vi "contrl.vi"() -> ()   [LabVIEW 2015]
uses:
  Ctrls/Main vari.ctl
  Mode/config/CHS.ctl
  Mode/config/singlechtype.ctl
  Ctrls/command.ctl
  TCPIP/TCPIP_enum.ctl
  TCPIP/TCPIPconfig.ctl
panel:
  out "P34 2":dbl
  in  "command":T1=22 items=["NO_Action", "start", "pause", "resum", "stop", "config", "System_constant", "7", "DAQ_init", "DAQ_config", "DAQ_start", "DAQ_read", "DAQ_stop", "DAQ_contrl", "14", "15", "16", "17", "18", "19", "Zsf_open", "Zsf_close", "Wkf_control", "Pump_switch", "dcf_switch", "JRQ_switch"]
  out "error out":errorcluster
  out "LED":bool[](array[boolean])
  in  "Tab Control":enum32{"核心舱", "实验舱", "温度曲线", "压力曲线", "内回路"}(tab)
  out "temp1 2":dbl(slide) caption="液温2" scale=0.0..100.0 scale format="%#_6f"
  out "temp2 2":dbl(slide) caption="液温1" scale=0.0..100.0 scale format="%.1f"
  out "PT22":dbl format="%#.1f"
  out "PT23":dbl
  out "转速":dbl format="%#.1f"
  out "流量计 2":dbl(knob) scale=0.0..1800.0 scale format="%#_6f"
  out "P34":dbl
  out "T4":dbl format="%#.1f"
  out "温控阀a":dbl(knob) scale=-10.0..60.0 scale format="%#.2f"
  out "zsf12":bool
  out "zsf11":bool
  out "zsf10":bool
  out "zsf9":bool
  out "zsf8":bool
  out "zsf7":bool
  out "zsf6":bool
  out "zsf5":bool
  out "zsf4":bool
  out "zsf3":bool
  out "zsf2":bool
  out "zsf1":bool
  in  "temctr_run 2":bool
  in  "temctr_value 2":dbl caption="设置"
  in  "temctr_type 2":enum16{"开度", "控温"}(ring)
  out "unit":string
  in  "temctr_run":bool
  in  "temctr_type":enum16{"开度", "控温"}(ring)
  in  "WP":bool
  in  "ZP":bool
  in  "rlmn 4":bool caption="加热模拟"
  in  "rlmn 3":bool caption="加热模拟"
  in  "rlmn 5":bool caption="加热模拟"
  out "PT21":dbl format="%#.1f"
  out "T2":dbl format="%#.1g"
  out "T22":dbl format="%#.1f"
  out "T1":dbl format="%#.1f"
  out "PT2":dbl format="%#.1f"
  out "T3":dbl format="%#.1f"
  out "T4":dbl format="%#.1f"
  out "PT3":dbl format="%#.1f"
  out "PT1":dbl format="%#.1f"
  out "P19":dbl format="%#.1f"
  out "P18":dbl format="%#.1f"
  out "P17":dbl format="%#.1g"
  out "P16":dbl format="%#.1f"
  out "P15":dbl format="%#.1f"
  out "P14":dbl format="%#.1f"
  out "P13":dbl format="%#.1f"
  out "P12":dbl format="%#.1f"
  out "DP2":dbl format="%#.2f"
  out "P11":dbl
  out "P10":dbl
  out "PT15":dbl
  out "PT16":dbl
  out "PT13":dbl
  out "PT14":dbl
  out "DP1":dbl format="%#.2g"
  out "P9":dbl format="%#.1f"
  out "P35":dbl format="%#.1f"
  out "P10":dbl format="%#.1f"
  out "P16":dbl format="%#.1f"
  out "P15":dbl format="%#.1f"
  out "P14":dbl format="%#.1f"
  out "P13":dbl format="%#.1f"
  out "P12":dbl format="%#.1f"
  out "P11":dbl format="%#.1f"
  out "T1":dbl format="%#.1f"
  out "PT8":dbl format="%#.1f"
  out "T2":dbl format="%#.1f"
  out "PT2":dbl format="%#.1f"
  out "PT1":dbl format="%#.2g"
  out "PT3":dbl format="%#.1f"
  out "T3":dbl format="%#.1f"
  out "PT4":dbl format="%#.1f"
  out "PT7":dbl format="%#.1f"
  out "PT9":dbl format="%#.1f"
  out "PT5":dbl format="%#.1f"
  out "ZF16":bool
  out "ZF17":bool
  in  "DCF19":bool
  in  "DCF18":bool
  in  "DCF17":bool
  in  "DCF16":bool
  in  "DCF15":bool
  in  "DCF14":bool
  in  "DCF13":bool
  in  "DCF12":bool
  in  "DCF11":bool
  in  "DCF10":bool
  in  "DCF9":bool
  in  "DCF8":bool
  out "DG8":bool
  out "DG7":bool
  out "DG6":bool
  out "DG5":bool
  out "G321":bool
  out "DG166":bool
  in  "qyflq 3":bool caption="气液分离器 3"
  out "ZF14":bool
  out "补偿器":dbl(slide) scale=0.0..200.0
  out "ZF13":bool
  out "G1114":bool
  out "G115":bool
  out "G131":bool
  out "G142":bool
  out "G112":bool
  out "G132":bool
  out "G133":bool
  out "G133":bool(c317)
  in  "DCF6":bool
  in  "DCF7":bool
  out "G113":bool
  in  "DCF5":bool
  out "G135":bool
  out "G134":bool
  out "G111":bool
  in  "DCF4":bool
  out "G141":bool
  out "流量计":dbl(knob) scale=0.0..1800.0 scale format="%#_6f"
  out "G181":bool
  out "G191":bool
  out "G201":bool
  out "补偿器":dbl(slide) scale=0.0..150.0 scale format="%#.1f"
  in  "DCF3":bool
  in  "DCF2":bool
  in  "DCF1":bool
  out "G999":bool
  out "G998":bool
  out "G401":bool
  out "G60":bool
  out "G58":bool
  out "G56":bool
  out "G53":bool
  out "G51":bool
  out "G49":bool
  out "G47":bool
  out "G45":bool
  out "G42":bool
  out "G61":bool
  out "G52":bool
  out "G54":bool
  out "G1313":bool
  out "G1312":bool
  out "G1311":bool
  out "G1310":bool
  out "G139":bool
  out "G138":bool
  out "G137":bool
  out "G136":bool
  in  "fsq6":bool caption="辐射器"
  in  "fsq5":bool caption="辐射器"
  in  "fsq4":bool caption="辐射器"
  in  "fsq3":bool caption="辐射器"
  in  "fsq2":bool caption="辐射器"
  out "G135":bool
  out "G134":bool
  out "G133":bool
  out "G132":bool
  out "G59":bool
  out "G57":bool
  out "G55":bool
  out "G43":bool
  out "G50":bool
  out "G48":bool
  out "G46":bool
  out "G44":bool
  out "G41":bool
  in  "ZSF12":bool
  in  "ZSF11":bool
  in  "ZSF10":bool
  in  "ZSF09":bool
  in  "ZSF08":bool
  in  "ZSF07":bool
  in  "ZSF06":bool
  in  "ZSF05":bool
  in  "ZSF04":bool
  in  "ZSF03":bool
  in  "ZSF02":bool
  out "G40":bool
  in  "ZSF01":bool
  in  "辐射器":bool
  out "电压":dbl
  out "电流":dbl
  out "转速":dbl
  out "DG11":bool
  out "ZF12":bool
  out "DG9":bool
  in  "DG4":bool
  in  "rlmn2":bool caption="加热模拟"
  out "DG3":bool
  in  "qyflq2":bool caption="气液分离器 2"
  out "ZF11":bool
  out "DG2":bool
  out "pumpD":bool
  out "ZG31":bool
  out "ZG14":bool
  out "ZF10":bool
  out "ZF9":bool
  out "ZF8":bool
  out "ZF7":bool
  out "ZF6":bool
  out "ZG8 2":bool
  out "ZF5":bool
  out "ZF4":bool
  out "ZF3":bool
  in  "qyflq":bool
  out "ZG8":bool
  out "ZF2":bool
  out "ZF1":bool
  out "ZG6":bool
  out "ZG30":bool
  out "ZG27":bool
  out "ZG24":bool
  out "ZG25":bool
  out "ZG26":bool
  out "ZG23":bool
  out "ZG22":bool
  out "ZG21":bool
  out "ZG20":bool
  out "ZG19":bool
  out "ZG18":bool
  out "ZG16":bool
  out "ZG15":bool
  out "ZG17":bool
  out "ZG13":bool
  in  "Zyshj":bool caption="视液镜"
  in  "ysj":bool caption="视液镜"
  out "ZG12":bool
  out "ZG11":bool
  out "ZG10":bool
  out "ZG9":bool
  out "ZG7":bool
  out "ZG5":bool
  out "ZG4":bool
  out "ZG3":bool
  out "ZG2":bool
  out "G38":bool
  out "ZG1":bool(c317)
  out "DG1":bool(c317)
  in  "rlmn１":bool caption="热量模拟"
  in  "yzmn":bool caption="液阻模拟"
  out "G37":bool
  out "G36":bool
  out "G34":bool
  out "G35":bool
  out "G30":bool(c317)
  out "温控阀ｂ":dbl(knob) scale=-10.0..60.0 scale format="%#.2g"
  out "G32":bool
  out "G31":bool
  out "SF2 2":bool
  out "G33":bool
  out "G29":bool
  out "G28":bool
  out "G27":bool
  out "temp1":dbl(slide) caption="液温2" scale=0.0..100.0 scale format="%#_6f"
  out "temp2":dbl(slide) caption="液温1" scale=0.0..100.0 scale format="%.1f"
  out "G25":bool
  out "G24":bool
  out "G23":bool
  out "G22":bool
  out "G21":bool
  out "G20":bool
  out "G19":bool
  out "G18":bool
  out "G17":bool
  out "G16":bool
  out "G15":bool
  out "G14":bool
  out "SF2":bool
  out "G13":bool
  out "pump":bool caption="外回路泵"
  out "G12":bool
  out "G11":bool
  out "G10":bool
  out "G9":bool
  out "G8":bool
  out "G7":bool
  out "G6":bool
  out "G4":bool
  out "G5":bool
  out "G3":bool
  out "pumpZ":bool caption="中温内回路泵"
  out "DG10":bool
  out "G2":bool
  out "SF1":bool
  out "wkf1":dbl caption="值" format="%#.1f"
  in  "temctr_value":dbl caption="设置"
  out "wkf2":dbl caption="值" format="%#.2g"
  out "temp1 4":dbl(slide) caption="液温2" scale=0.0..100.0 scale format="%#_6f"
  out "temp2 4":dbl(slide) caption="液温1" scale=0.0..100.0 scale format="%.1f"
  out "PT22 2":dbl format="%#.1f"
  out "PT23 2":dbl
  out "转速  3":dbl format="%#.1f"
  out "T4 3":dbl caption="T4" format="%#.1f"
  out "实验舱温控阀a":dbl(knob) caption="温控阀a" scale=-10.0..60.0 scale format="%#.2f"
  in  "temctr_run 4":bool
  in  "temctr_value 4":dbl caption="设置"
  in  "temctr_type 4":enum16{"开度", "控温"}(ring)
  out "unit 2":string
  in  "temctr_run 3":bool
  in  "temctr_type 3":enum16{"开度", "控温"}(ring)
  in  "WP 2":bool
  in  "ZP 2":bool
  in  "rlmn 8":bool caption="加热模拟"
  in  "rlmn 7":bool caption="加热模拟"
  in  "rlmn 6":bool caption="加热模拟"
  out "PT21 2":dbl format="%#.1f"
  out "T2 3":dbl format="%#.1g"
  out "T22 2":dbl format="%#.1f"
  out "T1 3":dbl format="%#.1f"
  out "PT2 3":dbl format="%#.1f"
  out "T3 3":dbl format="%#.1f"
  out "T4 2":dbl format="%#.1f"
  out "PT3 3":dbl format="%#.1f"
  out "PT1 3":dbl format="%#.1f"
  out "P19syc":dbl caption="内压传感器" format="%#.1f"
  out "P18 2":dbl format="%#.1f"
  out "P17 2":dbl format="%#.1g"
  out "P16 3":dbl format="%#.1f"
  out "P15 3":dbl format="%#.1f"
  out "P14 3":dbl format="%#.1f"
  out "P13 3":dbl format="%#.1f"
  out "P12 3":dbl format="%#.1f"
  out "DP2 2":dbl format="%#.2f"
  out "P11 3":dbl
  out "P10 3":dbl
  out "PT15 2":dbl
  out "PT16 2":dbl
  out "PT13 2":dbl
  out "PT14 2":dbl
  out "DP_syc":dbl caption="DP" format="%#.2g"
  out "syP9":dbl caption="外压2" format="%#.1f"
  out "syP35":dbl caption="外压3" format="%#.1f"
  out "P10_syc":dbl format="%#.1f"
  out "T1_syc":dbl caption="T1" format="%#.1f"
  out "PT8 2":dbl format="%#.1f"
  out "T2 2":dbl format="%#.1f"
  out "PT2 2":dbl format="%#.1f"
  out "PT1 2":dbl format="%#.2g"
  out "PT3 2":dbl format="%#.1f"
  out "T3 2":dbl format="%#.1f"
  out "PT4 2":dbl format="%#.1f"
  out "PT7 2":dbl format="%#.1f"
  out "PT9 2":dbl format="%#.1f"
  out "PT5 2":dbl format="%#.1f"
  out "ZF16 2":bool
  out "ZF17 2":bool
  out "DG8 2":bool
  out "DG7 2":bool
  out "DG6 2":bool
  out "DG5 2":bool
  out "G321 2":bool
  out "DG166 2":bool
  in  "qyflq 4":bool caption="气液分离器 3"
  out "ZF14 2":bool
  out "补偿器_sycw":dbl(slide) scale=0.0..200.0
  out "ZF13 2":bool
  out "G112 2":bool
  out "G132 3":bool
  out "G133 4":bool
  out "G133 3":bool(c317)
  out "G113 2":bool
  out "G135 3":bool
  out "G134 3":bool
  out "G111 2":bool
  out "G141 2":bool
  out "补偿器 2":dbl(slide) scale=0.0..150.0 scale format="%#.1f"
  out "G999 2":bool
  out "G998 2":bool
  out "G401 2":bool
  out "G60 2":bool
  out "G58 2":bool
  out "G56 2":bool
  out "G53 2":bool
  out "G51 2":bool
  out "G49 2":bool
  out "G47 2":bool
  out "G45 2":bool
  out "G42 2":bool
  out "G61 2":bool
  out "G52 2":bool
  out "G54 2":bool
  out "G1313 2":bool
  out "G1312 2":bool
  out "G1311 2":bool
  out "G1310 2":bool
  out "G139 2":bool
  out "G138 2":bool
  out "G137 2":bool
  out "G136 2":bool
  in  "fsq6 2":bool caption="辐射器"
  in  "fsq5 2":bool caption="辐射器"
  in  "fsq4 2":bool caption="辐射器"
  in  "fsq3 2":bool caption="辐射器"
  in  "fsq2 2":bool caption="辐射器"
  out "G135 2":bool
  out "G134 2":bool
  out "G133 2":bool
  out "G132 2":bool
  out "G59 2":bool
  out "G57 2":bool
  out "G55 2":bool
  out "G43 2":bool
  out "G50 2":bool
  out "G48 2":bool
  out "G46 2":bool
  out "G44 2":bool
  out "G41 2":bool
  out "G40 2":bool
  in  "辐射器 2":bool
  out "电压 2":dbl
  out "电流 2":dbl
  out "转速 2":dbl
  out "DG11 2":bool
  out "ZF12 2":bool
  out "DG9 2":bool
  in  "DG4 2":bool
  in  "rlmn2 2":bool caption="加热模拟"
  out "DG3 2":bool
  in  "qyflq2 2":bool caption="气液分离器 2"
  out "ZF11 2":bool
  out "DG2 2":bool
  out "pumpD 2":bool
  out "ZG31 2":bool
  out "ZG14 2":bool
  out "ZF10 2":bool
  out "ZF9 2":bool
  out "ZF8 2":bool
  out "ZF7 2":bool
  out "ZF6 2":bool
  out "ZG8 4":bool
  out "ZF5 2":bool
  out "ZF4 2":bool
  out "ZF3 2":bool
  in  "qyflq 2":bool
  out "ZG8 3":bool
  out "ZF2 2":bool
  out "ZF1 2":bool
  out "ZG6 2":bool
  out "ZG30 2":bool
  out "ZG27 2":bool
  out "ZG24 2":bool
  out "ZG25 2":bool
  out "ZG26 2":bool
  out "ZG23 2":bool
  out "ZG22 2":bool
  out "ZG21 2":bool
  out "ZG20 2":bool
  out "ZG19 2":bool
  out "ZG18 2":bool
  out "ZG16 2":bool
  out "ZG15 2":bool
  out "ZG17 2":bool
  out "ZG13 2":bool
  in  "Zyshj 2":bool caption="视液镜"
  in  "ysj 2":bool caption="视液镜"
  out "ZG12 2":bool
  out "ZG11 2":bool
  out "ZG10 2":bool
  out "ZG9 2":bool
  out "ZG7 2":bool
  out "ZG5 2":bool
  out "ZG4 2":bool
  out "ZG3 2":bool
  out "ZG2 2":bool
  out "G38 2":bool
  out "ZG1 2":bool(c317)
  out "DG1 2":bool(c317)
  in  "rlmn１ 2":bool caption="热量模拟"
  in  "yzmn 2":bool caption="液阻模拟"
  out "G37 2":bool
  out "G36 2":bool
  out "G34 2":bool
  out "G35 2":bool
  out "G30 2":bool(c317)
  out "温控阀ｂ 2":dbl(knob) scale=-10.0..60.0 scale format="%#.2g"
  out "G32 2":bool
  out "G31 2":bool
  out "SF2 4":bool
  out "G33 2":bool
  out "G29 2":bool
  out "G28 2":bool
  out "G27 2":bool
  out "temp1 3":dbl(slide) caption="液温2" scale=0.0..100.0 scale format="%#_6f"
  out "temp2 3":dbl(slide) caption="液温1" scale=0.0..100.0 scale format="%.1f"
  out "G25 2":bool
  out "G24 2":bool
  out "G23 2":bool
  out "G22 2":bool
  out "G21 2":bool
  out "G20 2":bool
  out "G19 2":bool
  out "G18 2":bool
  out "G17 2":bool
  out "G16 2":bool
  out "G15 2":bool
  out "G14 2":bool
  out "SF2 3":bool
  out "G13 2":bool
  out "pump 2":bool caption="外回路泵"
  out "G12 2":bool
  out "G11 2":bool
  out "G10 2":bool
  out "G9 2":bool
  out "G8 2":bool
  out "G7 2":bool
  out "G6 2":bool
  out "G4 2":bool
  out "G5 2":bool
  out "G3 2":bool
  out "pumpZ 2":bool caption="中温内回路泵"
  out "DG10 2":bool
  out "G2 2":bool
  out "SF1 2":bool
  out "wkf1 2":dbl caption="值" format="%#.1f"
  in  "temctr_value 3":dbl caption="设置"
  out "wkf2 2":dbl caption="值" format="%#.2g"
  out "测试数据":string[][](table)
  out "T Wave":dbl[](graph) caption="Vibr Wave"
  out "XY Graph":cluster{cluster{"time":dbl, "Y":dbl}[]}[](graph)
  out "Vibr Wave 3":dbl[](graph) caption="Vibr Wave"
  out "triger?":bool caption="采集\n触发"
  out "save":bool caption="数据\n存储"
  in  "Query":bool
  in  "Exit":bool
  in  "Acquire":bool
  in  "Config":bool
  in  "Vibr Waveform 2":waveform(dbl)[](array[waveform])
  out "throber 2":bool
  in  "Main Vari":T2={"Error"={"status"=FALSE, "code"=0, "source"=""}, "Test Info"={"Test Name"="", "Tester"=""}, "StateName"="", "Display Info"=[{"Frequency"=0.0, "RMS"=0.0}, {"Frequency"=0.0, "RMS"=0.0}, {"Frequency"=0.0, "RMS"=0.0}, {"Frequency"=0.0, "RMS"=0.0}, {"Frequency"=0.0, "RMS"=0.0}], "粉尘特性"={"名称"="", "粒径"="", "含水量"=""}, "测试条件"={"初始含氧量"="", "初始压力"="", "测试浓度"="", "点火能量"="", "初始温度"="", "反应器体积[L]"=0.0}, "ch size"=0, "data out"=[], "CHS"=[], "CalData"=[]} {"CHS"."display" format="%b"}
  # "流体回路多回路试验平台测试系统"
  # "Measurement System Ver 1.0  Copyright  by M_tech design studio"
  # "温控阀控制"
  # "液视镜"
  # "温控阀控制"
  # "液视镜"
  # "通道名称"
  # "颜色"
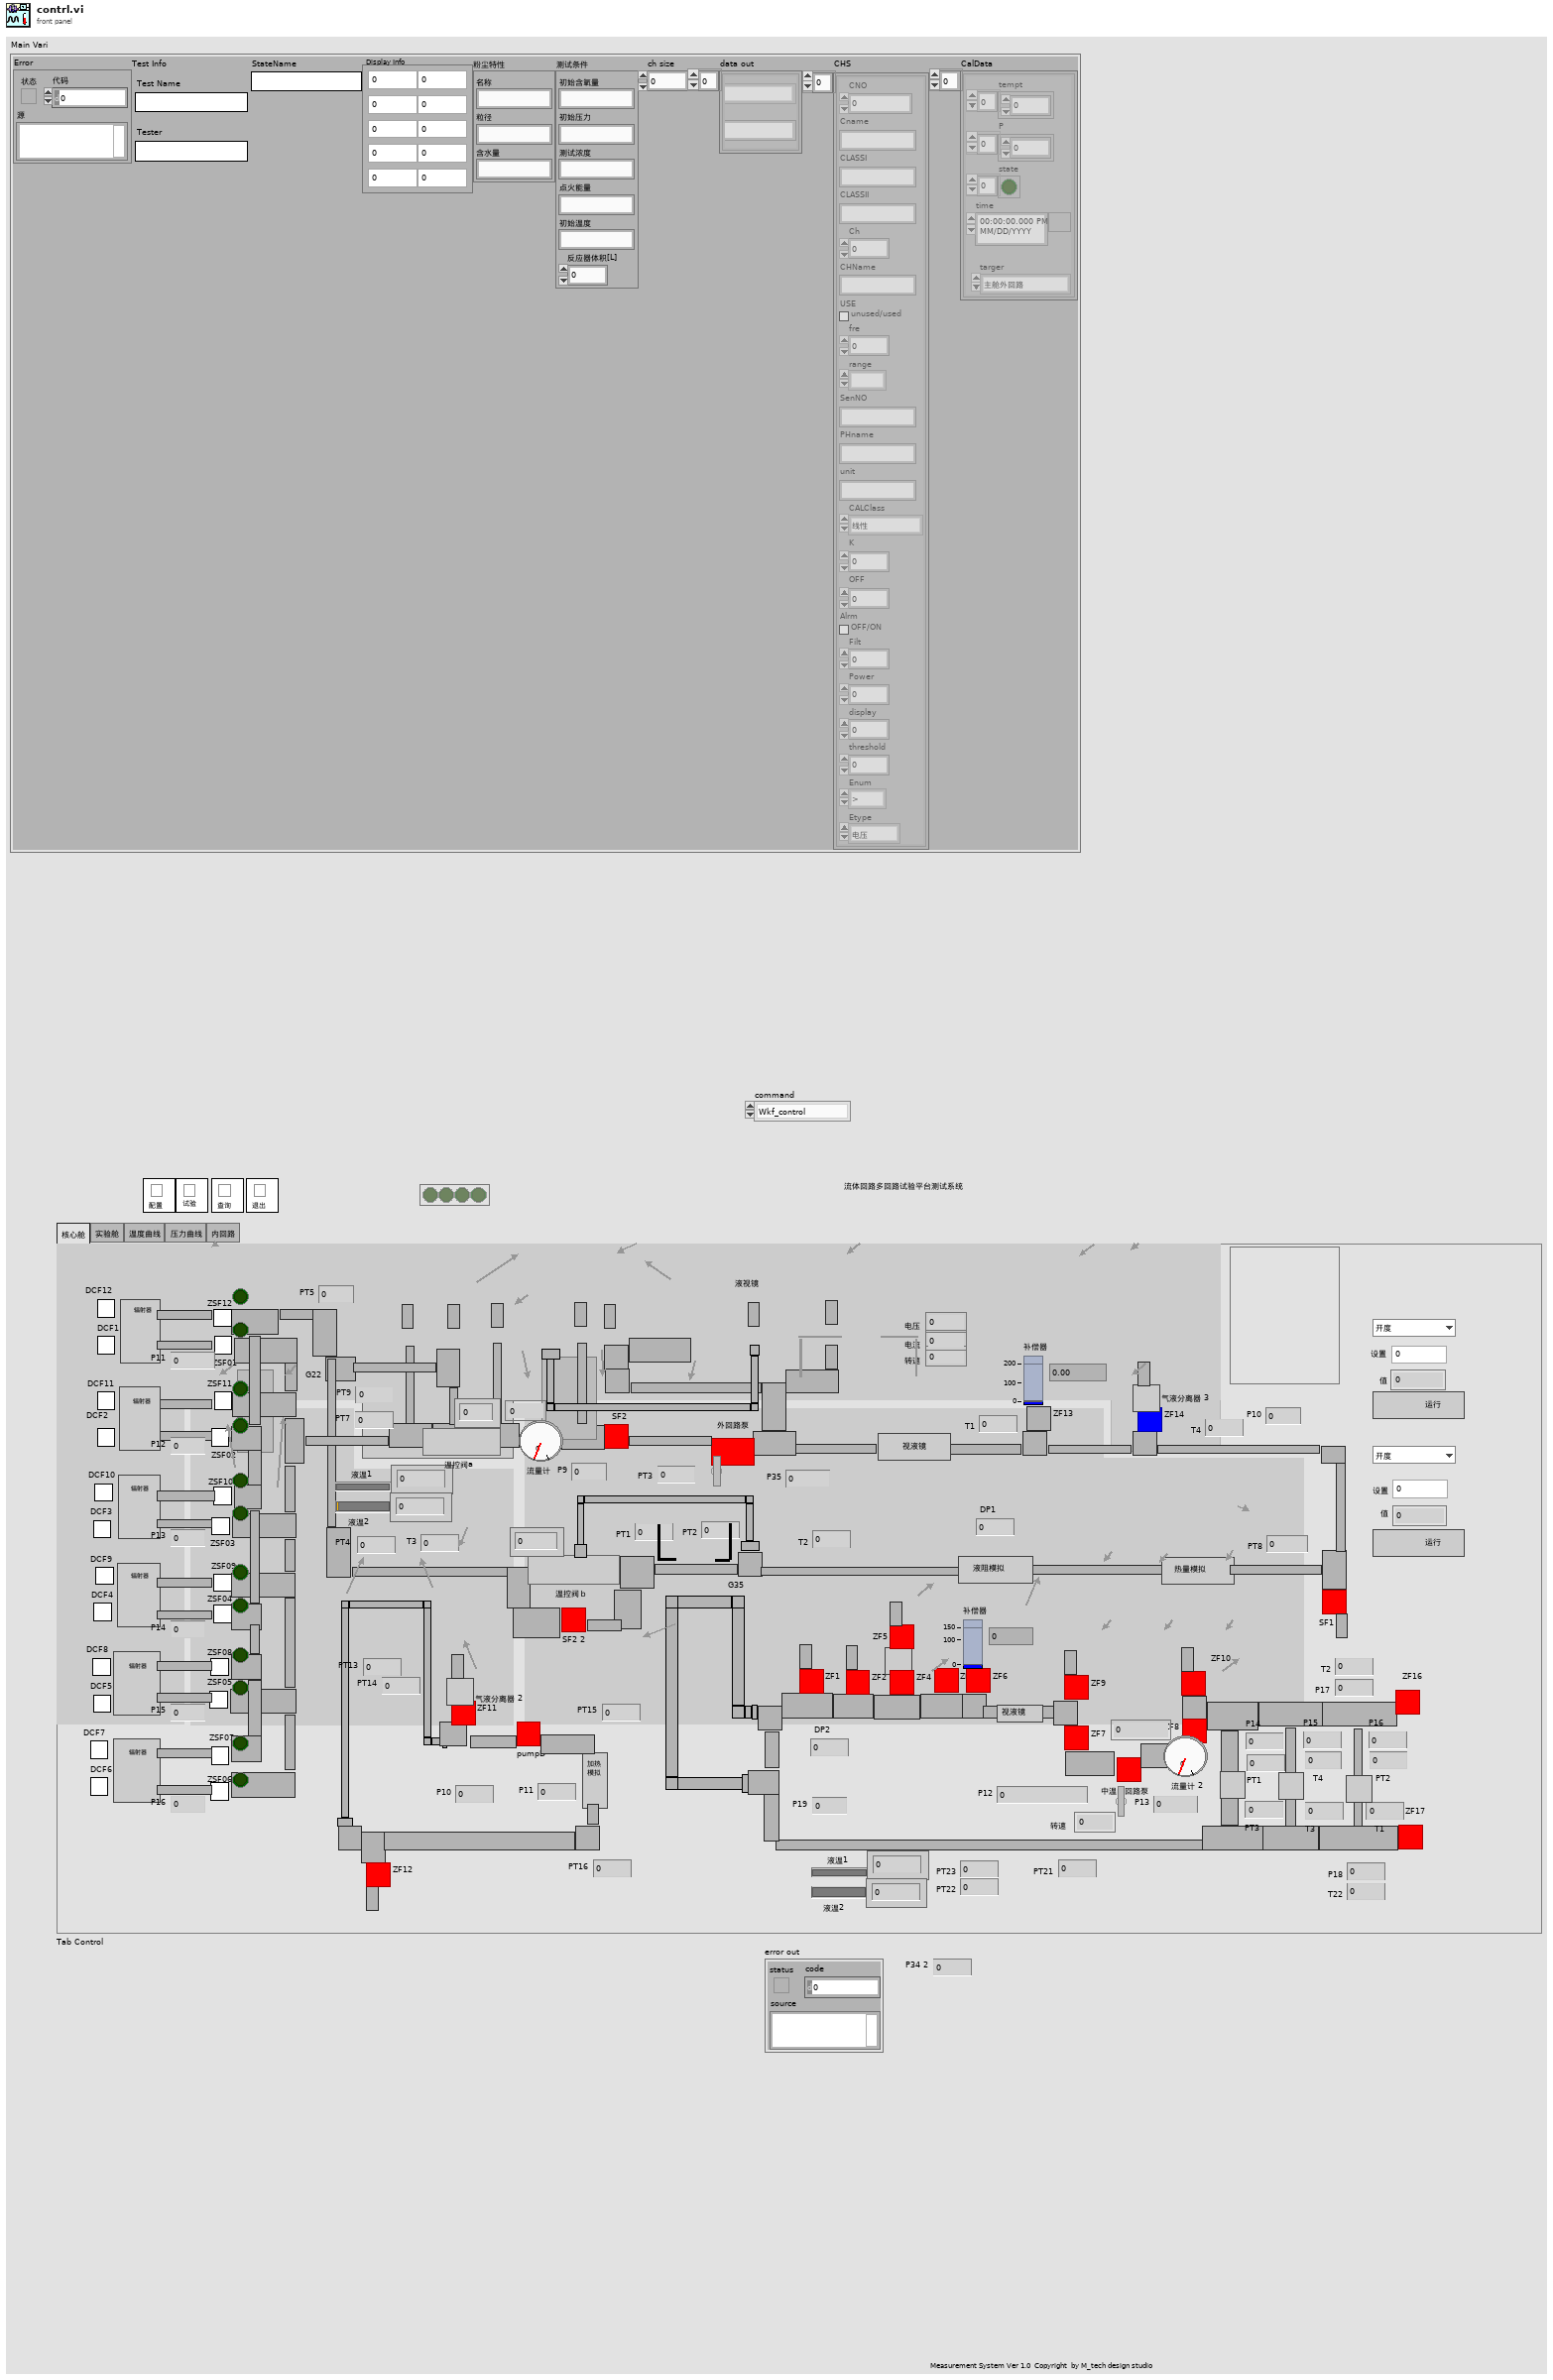
[diagram p1: front panel]
types:
  T1 = typedef "command.ctl" = u16
  T2 = typedef "Main vari.ctl" = cluster{"Error":errorcluster, "Test Info":cluster{"Test Name":string, "Tester":string}, "StateName":string, "Display Info":T3, "粉尘特性":T4, "测试条件":T5, "ch size":u8, "data out":cluster{"targer":enum16{"主舱外回路", "主舱内回路", "实验舱外回路", "实验舱内回路"}, "data":string}[], "CHS":T6, "CalData":cluster{"tempt":dbl[], "P":dbl[], "state":bool[], "time":timestamp, "targer":enum16{"主舱外回路", "主舱内回路", "实验舱外回路", "实验舱内回路"}}[]}
  T3 = typedef "Display Information_Ctrls-某型振动实验台测试系统.ctl" = cluster{"Frequency":dbl, "RMS":dbl}[]
  T4 = typedef "粉尘特性.ctl" = cluster{"名称":string, "粒径":string, "含水量":string}
  T5 = typedef "测试条件.ctl" = cluster{"初始含氧量":string, "初始压力":string, "测试浓度":string, "点火能量":string, "初始温度":string, "反应器体积[L]":dbl}
  T6 = typedef "CHS.ctl" = T7[]
  T7 = typedef "singlechtype.ctl" = cluster{"CNO":u8, "Cname":string, "CLASSI":string, "CLASSII":string, "Ch":u8, "CHName":string, "USE":bool, "fre":dbl, "range":enum16{""}, "SenNO":string, "PHname":string, "unit":string, "CALClass":enum8{"线性", "查表", "公式"}, "K":dbl, "OFF":dbl, "Alrm":bool, "Filt":dbl, "Power":u8, "display":u8, "threshold ":dbl, "Enum":enum16{">", ">=", "<", "<=", "<>(在范围内）", "><（在范围外）"}, "Etype":enum16{"电压", "电流", "电阻", "热电偶K", "热电偶T"}}
  T8 = typedef "Enum queue_Ctrls-某型振动实验台测试系统.ctl" = enum16{"Noop", "Send Pro1", "Send data", "Get Pro1", "Get data", "Flush Pro1", "Flush data", "Destroy Pro1", "Destroy data"}
  T9 = typedef "TCPIPconfig.ctl" = cluster{"add":string, "port":u32, "timeout":u16, "connection ID":refnum<k5>, "targer":enum16{"主舱外回路", "主舱内回路", "实验舱外回路", "实验舱内回路"}}[]
  T10 = cluster{"targer":enum16{"主舱外回路", "主舱内回路", "实验舱外回路", "实验舱内回路"}, "data":string}[]
  T11 = cluster{"targer":enum16{"主舱外回路", "主舱内回路", "实验舱外回路", "实验舱内回路"}, "data":string}
  T12 = typedef "TCPIP_enum.ctl" = enum16{"init", "connect", "command", "write", "read", "close", "null"}
  T13 = cluster{"T":cluster{"TSlop":dbl[], "T0":dbl[]}, "P":cluster{"P0":dbl[], "Pslop":dbl[]}}[]
  T14 = cluster{"T":cluster{"index":dbl, "name":string, "unit":string, "代号":string}[], "P":cluster{"index":dbl, "name":string, "unit":string, "代号":string}[], "state":cluster{"index":dbl, "name":string, "unit":string, "代号":string}[], "time":timestamp, "targer":enum16{"主舱外回路", "主舱内回路", "实验舱外回路", "实验舱内回路"}}[]
  T15 = enum16{"init", "trig", "save", "stop", "Default"}
  T16 = typedef "Enum File IO - FGV(V)_Ctrls-某型振动实验台测试系统.ctl" = enum16{"New", "Open", "Write Info", "Write Data", "Read Info", "Read Chan Names", "Read Data", "Close", "None"}
  T17 = cluster{"tempt":dbl[], "P":dbl[], "state":bool[], "time":timestamp, "targer":enum16{"主舱外回路", "主舱内回路", "实验舱外回路", "实验舱内回路"}}[]
  T18 = cluster{"tempt":dbl[], "P":dbl[], "state":bool[], "time":timestamp, "targer":enum16{"主舱外回路", "主舱内回路", "实验舱外回路", "实验舱内回路"}}
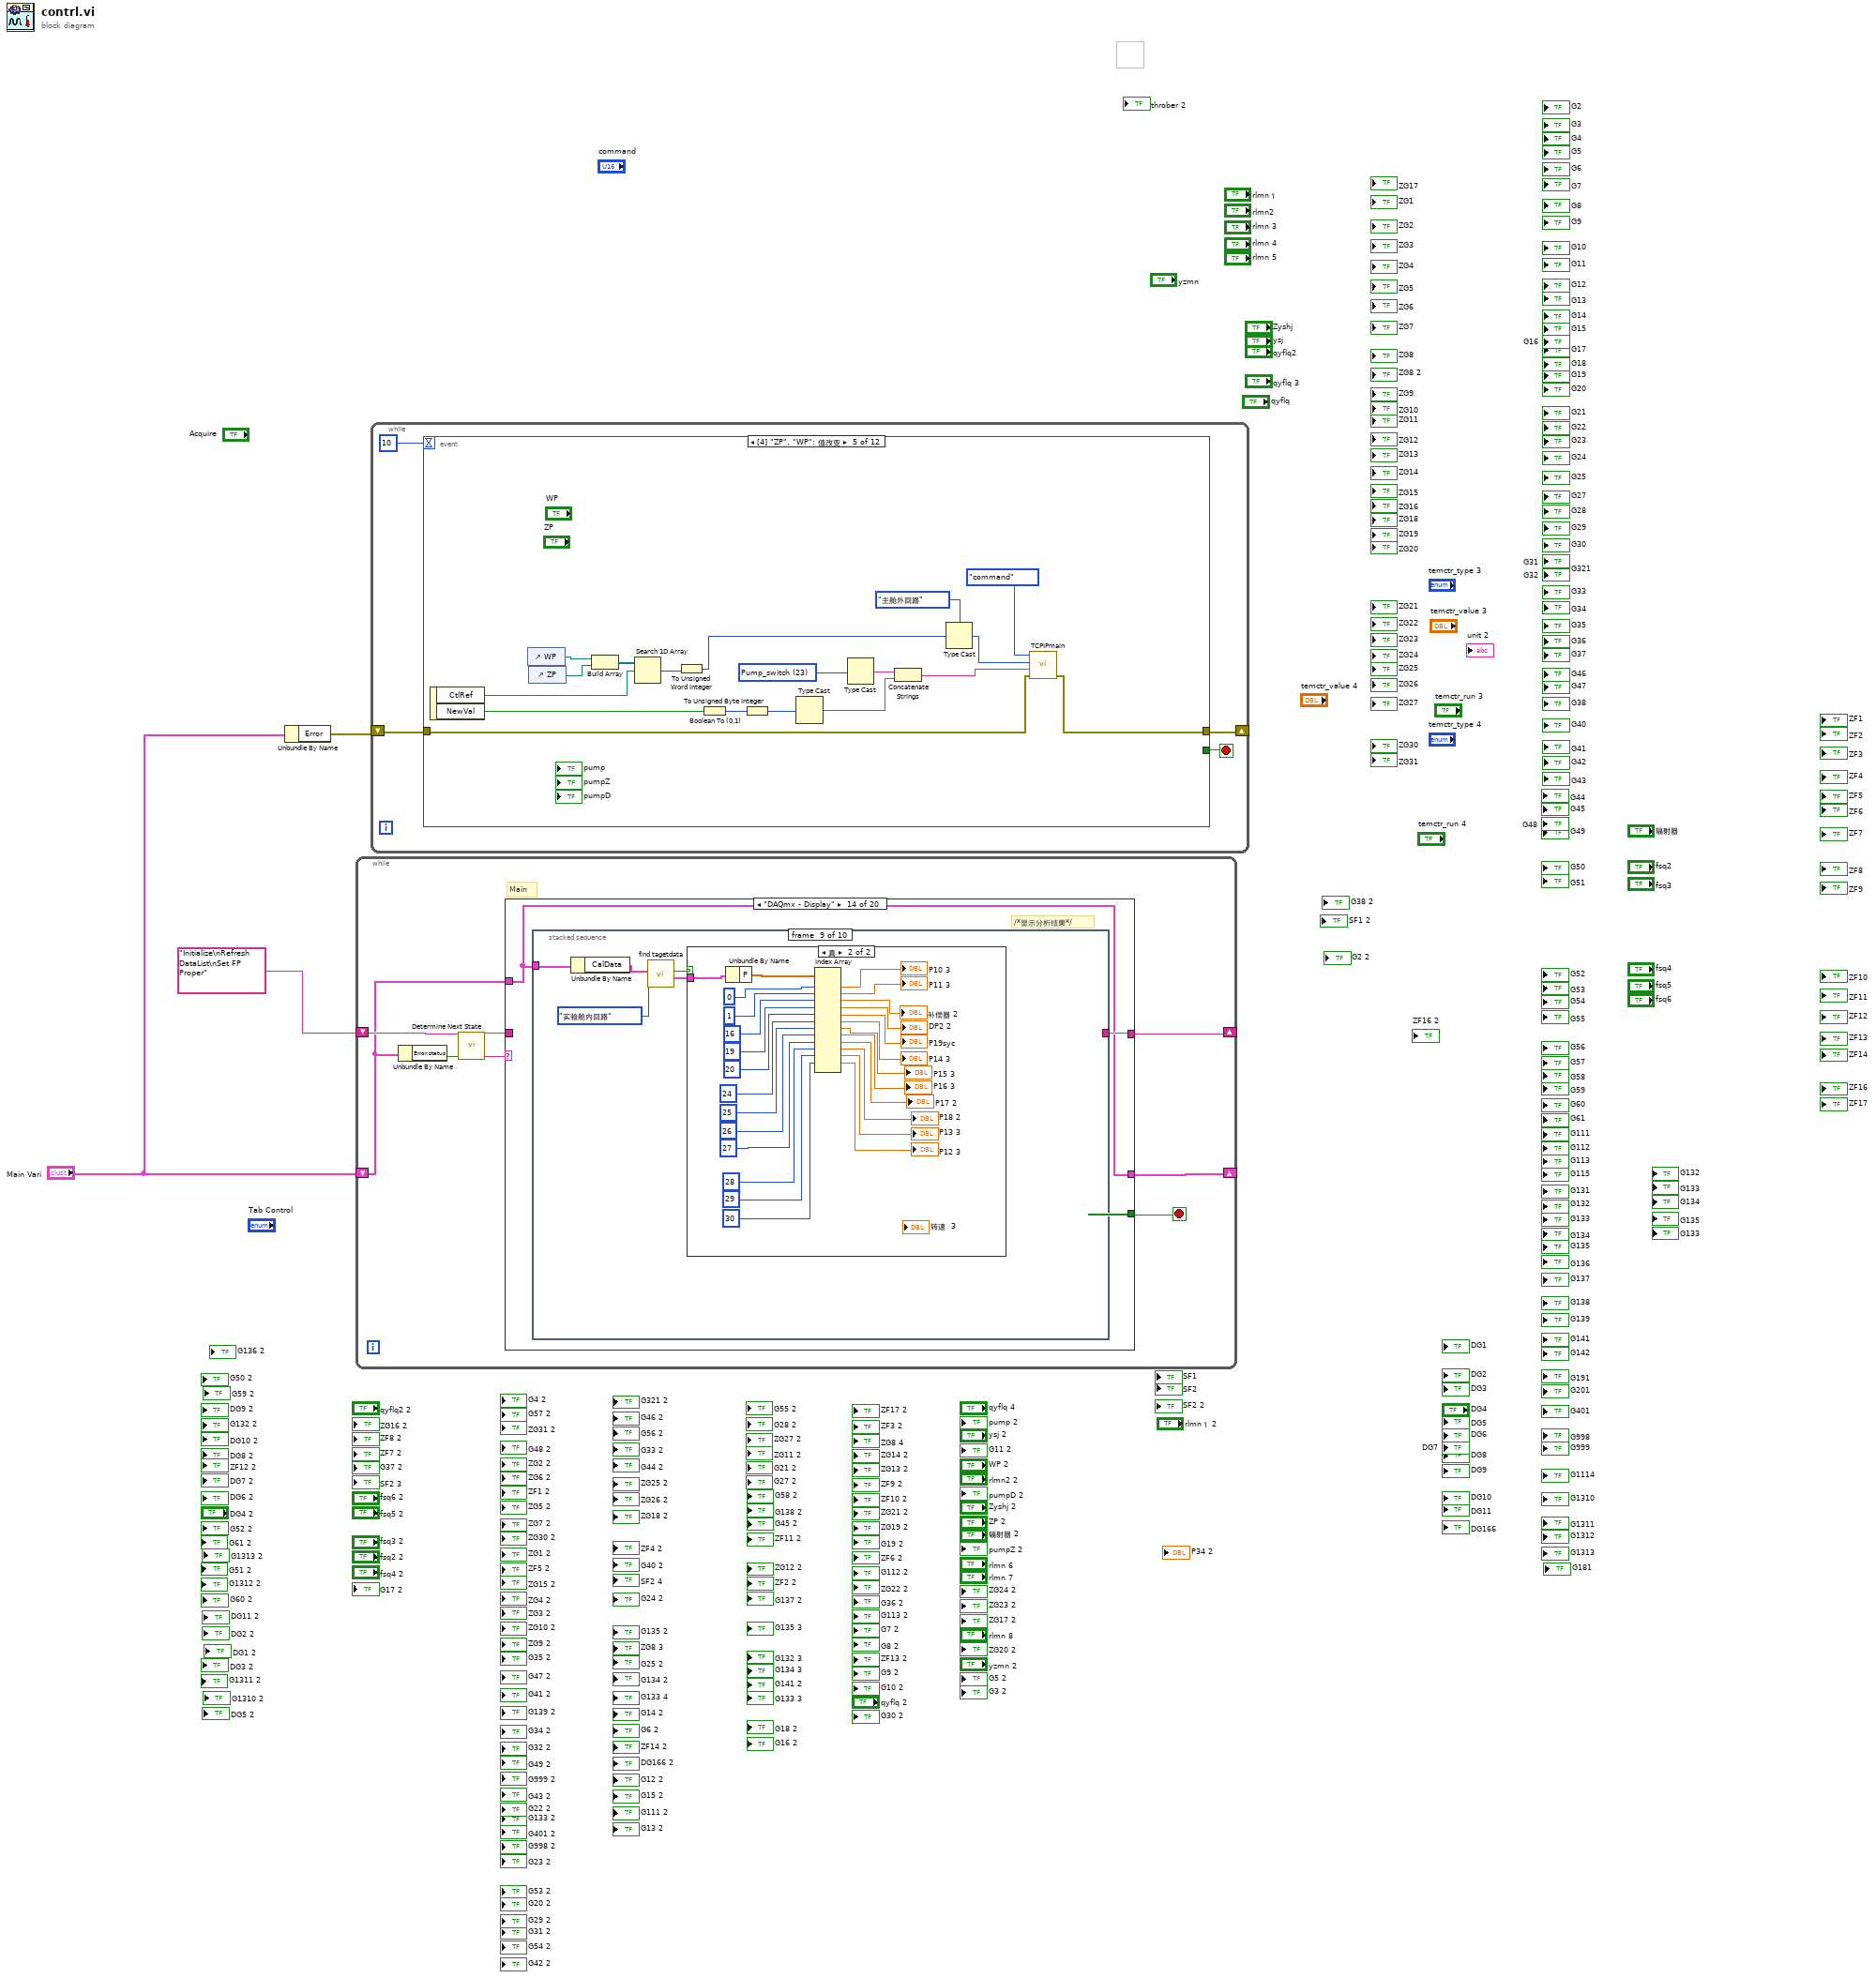
[diagram p0: block diagram]
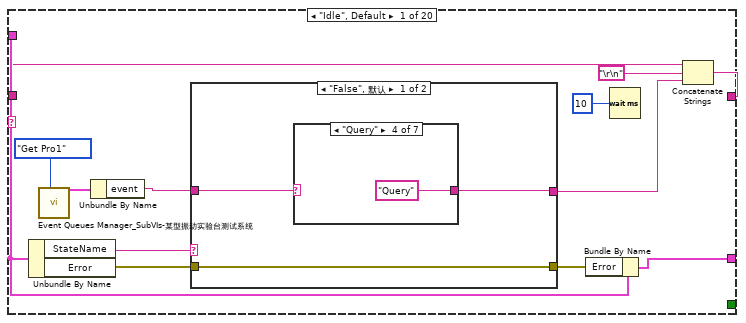
[diagram p2: hidden frame]
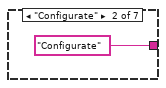
[diagram p4: hidden frame]
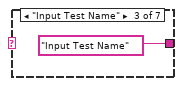
[diagram p5: hidden frame]
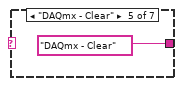
[diagram p6: hidden frame]
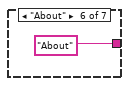
[diagram p7: hidden frame]
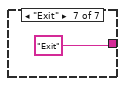
[diagram p8: hidden frame]
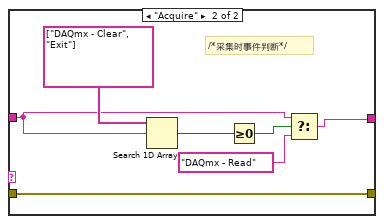
[diagram p9: hidden frame]
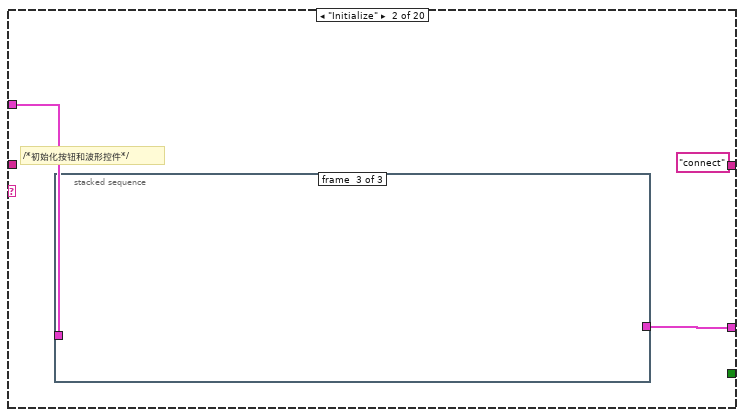
[diagram p10: hidden frame]
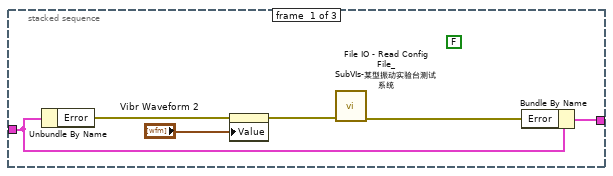
[diagram p11: hidden frame]
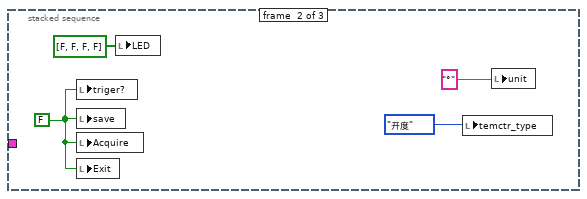
[diagram p12: hidden frame]
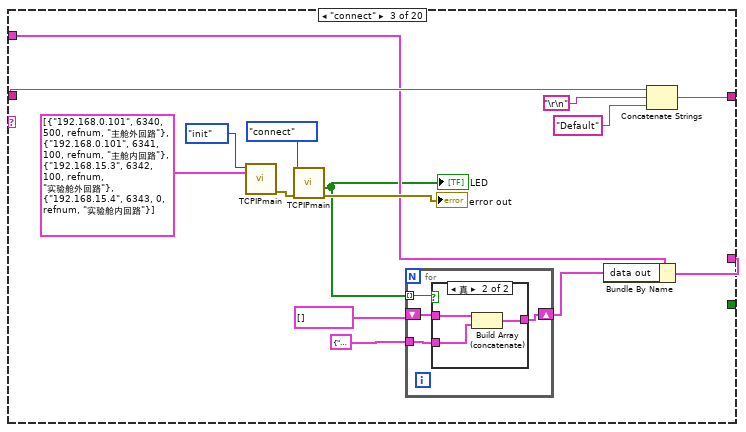
[diagram p13: hidden frame]
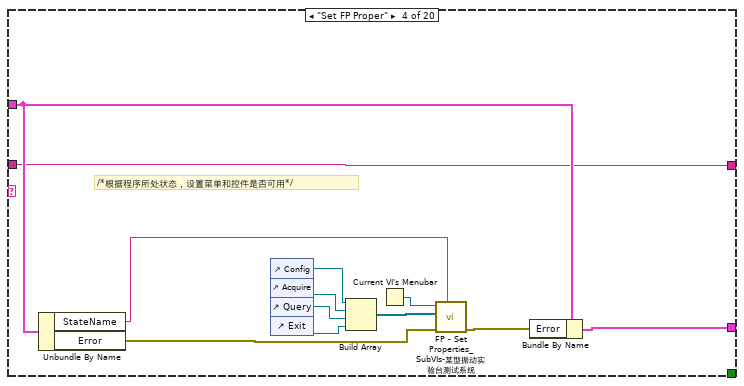
[diagram p15: hidden frame]
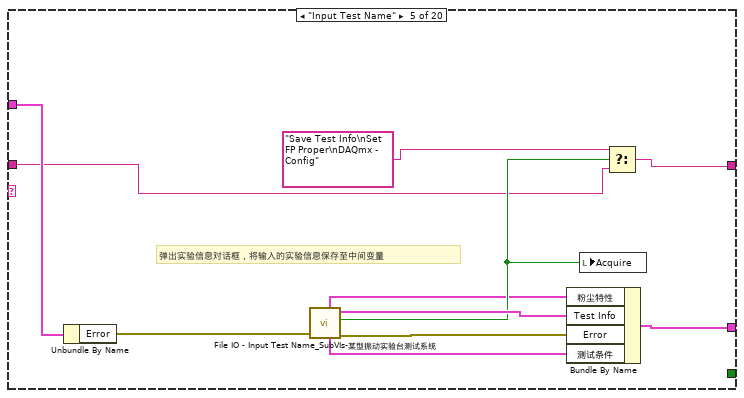
[diagram p16: hidden frame]
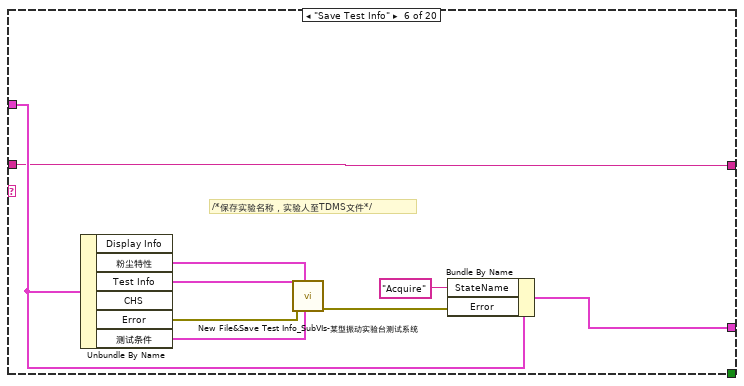
[diagram p17: hidden frame]
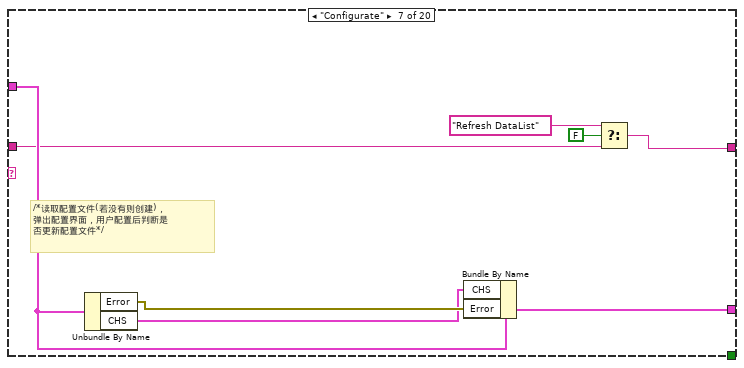
[diagram p18: hidden frame]
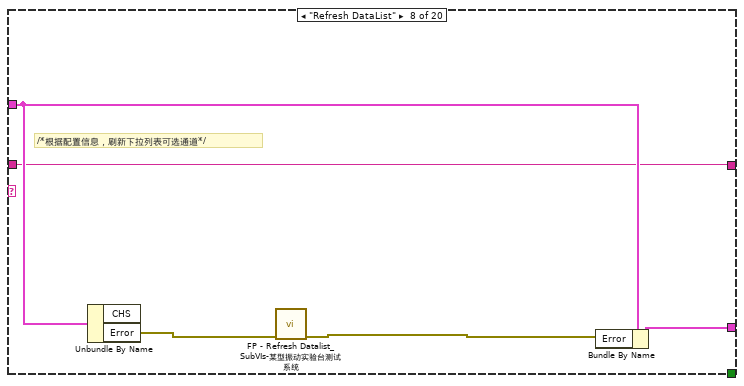
[diagram p19: hidden frame]
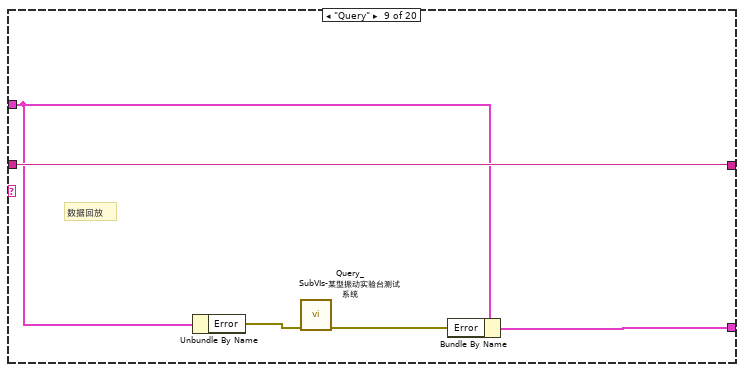
[diagram p20: hidden frame]
diagram:
  n1 = Unbundle By Name("Main Vari") -> ("Error"=w1:errorcluster)
  n2 = while {
    shift-right: [w10] -> _
    shift-left: "Main Vari" -> [w6]
    shift-right: [w8] -> _
    shift-left: "Initialize\nRefresh DataList\nSet FP Proper" ("Previous State") -> [w9]
    stop <- w11 stop-if-true
    # "Main"
    n3 = Unbundle By Name(w6) -> ("Error.status"=w5:bool)
    n4 = call "Determine Next State.vi"("Status?"=w5, "Previous State"=w9) -> ("New State"=w4:string, "Remaining States"=w7:string)  [unwired: 4 out]
    n5 = case shown="\"DAQmx - Display\"" w4 {
      tunnel: [_ _ _ _ _ _ _ _ _ _ _ _ _ _ _ _ _ _ _ TRUE] -> w11
      tunnel: w6 -> [w18 w43 w59 w80 w96 w107 w117 w121 w124 w129 w141 w149 w162 w165 w436 w451 w460 w466 w471 w474]
      tunnel: [w17 w44 w60 w79 w95 w106 w116 w120 w123 w129 w143 w152 w161 w165 w436 w457 w460 w465 w470 w473] -> w10
      tunnel: [w14 "connect" ("Remaining States") w64 w78 w92 w105 w115 w119 w127 w128 "DAQmx - Read" ("event") w155 "DAQmx - Display" ("event") w166 "Idle" ("Remaining States") "Set FP Proper" ("Remaining States") w461 w462 w469 w472] -> w8
      tunnel: w7 -> [w15 _ w63 w78 w94 w105 w113 w119 w127 w128 _ _ _ _ _ _ w461 w462 w469 w472]
      frame "Idle", Default {
        n6 = Unbundle By Name(w18) -> ("StateName"=w20:string, "Error"=w19:errorcluster)
        n7 = call "Event Queues Manager_SubVIs-某型振动实验台测试系统.vi"("Mode"=Enum_queue_Ctrls-某型振动实验台测试系统."Get Pro1" ("Mod")) -> ("Process1"=w23:cluster{"event":string, "Message":variant})  [unwired: 4 in, 6 out]
        n8 = Unbundle By Name(w23) -> ("event"=w21:string)
        n9 = case shown="\"False\", 默认" w20 {
          tunnel: w21 -> [w27 w38]
          tunnel: [w26 w37] -> w13
          tunnel: w19 -> [w25 w36]
          tunnel: [w25 w36] -> w16
          frame "False", Default {
            n10 = case shown="\"Query\"" w27 {
              selector: w27 -> [w28 _ _ _ _ _ _]
              tunnel: [w28 "Configurate" ("Previous State") "Input Test Name" ("event") "Query" ("event") "DAQmx - Clear" ("event") "About" ("event") "Exit" ("event")] -> w26
              frame "Idle", Default {
              }
              frame "Configurate" {
              }
              frame "Input Test Name" {
              }
              frame "Query" {
              }
              frame "DAQmx - Clear" {
              }
              frame "About" {
              }
              frame "Exit" {
              }
            }
          }
          frame "Acquire" {
            # "/*采集时事件判断*/"
            n11 = Search 1D Array(1D array=string[] ["DAQmx - Clear", "Exit"], element=w38) -> (index of element=w40:i32)  [unwired: 1 out]
            n12 = Greater Or Equal To 0?(x=w40) -> (x >= 0?=w39:bool)
            n13 = Select(t=w38, s=w39, f="DAQmx - Read" ("event")) -> (s? t:f=w37:string)
          }
        }
        n14 = Bundle By Name(cluster=w18, "Error"=w16) -> (w17:T2)
        n15 = Wait (ms)(milliseconds to wait=u32 10) -> ()  [unwired: 1 out]
        n16 = Concatenate Strings(w15, "\r\n", w13) -> (w14:string)
      }
      frame "Initialize" {
        # "/*初始化按钮和波形控件*/"
        n17 = stacked-sequence {
          tunnel: [w49 _ _] -> w44
          tunnel: w43 -> [w45 _ _]
          frame #0 {
            (unwired) FALSE ("Task Info.Accele.Simulate")
            n18 = Unbundle By Name(w45) -> ("Error"=w48:errorcluster)
            n19 = property on="T Wave" class="WFGraph (严格)"(error in=w48, "Value"="Vibr Waveform 2") -> (error out=w47:errorcluster)  [unwired: 1 in, 1 out]
            n20 = call "File IO - Read Config File_SubVIs-某型振动实验台测试系统.vi"("Error In"=w47) -> ("Error Out"=w46:errorcluster)  [unwired: 8 out]
            n21 = Bundle By Name(cluster=w45, "Error"=w46) -> (w49:T2)
          }
          frame #1 {
            w54 = FALSE ("Start")
            n22 = local write "triger?"(w54) -> ()
            n23 = local write "save"(w54) -> ()
            n24 = local write "Acquire"(w54) -> ()
            n25 = local write "Exit"(w54) -> ()
            n26 = local write "LED"(bool[] [FALSE, FALSE, FALSE, FALSE] ("LED")) -> ()
            n27 = local write "temctr_type"(enum16{"开度", "控温"}."开度" ("temctr_type")) -> ()
            n28 = local write "unit"("°") -> ()
          }
          frame #2 {
          }
        }
      }
      frame "connect" {
        n29 = call "TCPIPmain.vi"("config"=T9 [{"add"="192.168.0.101", "port"=6340, "timeout"=500, "connection ID"=refnum, "targer"=enum."主舱外回路"}, {"add"="192.168.0.101", "port"=6341, "timeout"=100, "connection ID"=refnum, "targer"=enum."主舱内回路"}, {"add"="192.168.15.3", "port"=6342, "timeout"=100, "connection ID"=refnum, "targer"=enum."实验舱外回路"}, {"add"="192.168.15.4", "port"=6343, "timeout"=0, "connection ID"=refnum, "targer"=enum."实验舱内回路"}], "Enum"=TCPIP_enum."init") -> ("error out"=w67:errorcluster)  [unwired: 6 in, 3 out]
        n30 = call "TCPIPmain.vi"("error in"=w67, "Enum"=TCPIP_enum."connect") -> ("error out"=→"error out":errorcluster, "LED"=w58:bool[])  [unwired: 6 in, 2 out]
        "LED" <- w58
        n31 = for {
          tunnel: w58 -> [w73] mode=indexing
          shift-right: [w70] -> w56
          shift-left: T10 [] ("data out") -> [w72]
          tunnel: T11 {"targer"=enum."主舱外回路", "data"=""} ("data out") -> [w71]
          n32 = case shown="真" w73 {
            tunnel: w72 -> [w74 w77]
            tunnel: w71 -> [_ w76]
            tunnel: [w74 w75] -> w70
            frame False {
            }
            frame True {
              n33 = Build Array (concatenate)(w77, w76) -> (w75:T10)
            }
          }
        }
        n34 = Bundle By Name(cluster=w59, "data out"=w56) -> (w60:T2)
        n35 = Concatenate Strings(w63, "\r\n", "Default" ("string")) -> (w64:string)
      }
      frame "Set FP Proper" {
        # "/*根据程序所处状态，设置菜单和控件是否可用*/"
        n36 = Unbundle By Name(w80) -> ("StateName"=w81:string, "Error"=w84:errorcluster)
        n37 = control-ref of="Config"() -> (w86:refnum<vi>)
        n38 = control-ref of="Acquire"() -> (w87:refnum<vi>)
        n39 = control-ref of="Query"() -> (w88:refnum<vi>)
        n40 = control-ref of="Exit"() -> (w89:refnum<vi>)
        n41 = Build Array(w86, w87, w88, w89) -> (w82:refnum<vi>[])
        n42 = Current VI's Menubar() -> (w85:refnum<k9>)
        n43 = call "FP - Set Properties_SubVIs-某型振动实验台测试系统.vi"("StateName"=w81, "error in (no error)"=w84, "Controls"=w82, "menu ref"=w85) -> ("error out"=w83:errorcluster)  [unwired: 7 out]
        n44 = Bundle By Name(cluster=w80, "Error"=w83) -> (w79:T2)
      }
      frame "Input Test Name" {
        # "弹出实验信息对话框，将输入的实验信息保存至中间变量"
        n45 = Unbundle By Name(w96) -> ("Error"=w97:errorcluster)
        n46 = call "File IO - Input Test Name_SubVIs-某型振动实验台测试系统.vi"("Error In"=w97) -> ("Error Out"=w98:errorcluster, "OK"=w99:bool, "Test Information"=w100:cluster{"Test Name":string, "Tester":string}, "测试条件"=w91:T5, "粉尘特性"=w90:T4)  [unwired: 6 out]
        n47 = Bundle By Name(cluster=w96, "粉尘特性"=w90, "Test Info"=w100, "Error"=w98, "测试条件"=w91) -> (w95:T2)
        n48 = local write "Acquire"(w99) -> ()
        n49 = Select(t="Save Test Info\nSet FP Proper\nDAQmx - Config", s=w99, f=w94) -> (s? t:f=w92:string)
      }
      frame "Save Test Info" {
        # "/*保存实验名称，实验人至TDMS文件*/"
        n50 = Unbundle By Name(w107) -> ("粉尘特性"=w103:T4, "Test Info"=w109:cluster{"Test Name":string, "Tester":string}, "Error"=w101:errorcluster, "测试条件"=w102:T5)  [unwired: 2 out]
        n51 = call "New File&Save Test Info_SubVIs-某型振动实验台测试系统.vi"("测试条件"=w102, "粉尘特性"=w103, "error in"=w101, "Test Info"=w109) -> ("error out"=w108:errorcluster)  [unwired: 1 in, 6 out]
        n52 = Bundle By Name(cluster=w107, "StateName"="Acquire", "Error"=w108) -> (w106:T2)
      }
      frame "Configurate" {
        # "/*读取配置文件(若没有则创建)，\n弹出配置界面，用户配置后判断是\n否更新配置文件*/"
        n53 = Unbundle By Name(w117) -> ("Error"=w112:errorcluster, "CHS"=w111:T6)
        n54 = Bundle By Name(cluster=w117, "CHS"=w111, "Error"=w112) -> (w116:T2)
        n55 = Select(t="Refresh DataList" ("f"), s=FALSE, f=w113) -> (s? t:f=w115:string)
      }
      frame "Refresh DataList" {
        # "/*根据配置信息，刷新下拉列表可选通道*/"
        n56 = Unbundle By Name(w121) -> ("Error"=w122:errorcluster)  [unwired: 1 out]
        n57 = call "FP - Refresh Datalist_SubVIs-某型振动实验台测试系统.vi"("error in"=w122) -> ("error out"=w118:errorcluster)  [unwired: 2 in, 8 out]
        n58 = Bundle By Name(cluster=w121, "Error"=w118) -> (w120:T2)
      }
      frame "Query" {
        # "数据回放"
        n59 = Unbundle By Name(w124) -> ("Error"=w126:errorcluster)
        n60 = call "Query_SubVIs-某型振动实验台测试系统.vi"("Error"=w126) -> ("Error"=w125:errorcluster)  [unwired: 10 out]
        n61 = Bundle By Name(cluster=w124, "Error"=w125) -> (w123:T2)
      }
      frame "-----------------" {
      }
      frame "DAQmx - Config" {
        w132 = T1 8 items=["NO_Action", "start", "pause", "resum", "stop", "config", "System_constant", "7", "DAQ_init", "DAQ_config", "DAQ_start", "DAQ_read", "DAQ_stop", "DAQ_contrl", "14", "15", "16", "17", "18", "19", ""] ("command")
        w138 = T1 10 items=["NO_Action", "start", "pause", "resum", "stop", "config", "System_constant", "7", "DAQ_init", "DAQ_config", "DAQ_start", "DAQ_read", "DAQ_stop", "DAQ_contrl", "14", "15", "16", "17", "18", "19", ""] ("command")
        w136 = T1 9 items=["NO_Action", "start", "pause", "resum", "stop", "config", "System_constant", "7", "DAQ_init", "DAQ_config", "DAQ_start", "DAQ_read", "DAQ_stop", "DAQ_contrl", "14", "15", "16", "17", "18", "19", ""] ("command")
        w130 = TCPIP_enum."write" ("Enum")
        n62 = Unbundle By Name(w141) -> ("Error"=w134:errorcluster)
        n63 = Type Cast(x=w132) -> (*(type *) &x=w131:string)  [unwired: 1 in]
        n64 = call "TCPIPmain.vi"("error in"=w134, "data in"=w131, "Enum"=w130) -> ("error out"=w133:errorcluster)  [unwired: 5 in, 3 out]
        n65 = Type Cast(x=w136) -> (*(type *) &x=w135:string)  [unwired: 1 in]
        n66 = call "TCPIPmain.vi"("error in"=w133, "data in"=w135, "Enum"=w130) -> ("error out"=w144:errorcluster)  [unwired: 5 in, 3 out]
        n67 = Unbundle By Name(w141) -> ("CHS"=w142:T6)
        n68 = call "chs_to_Netdata.vi"("CHS"=w142) -> ("ChString"=w145:string)  [unwired: 8 in]
        n69 = call "TCPIPmain.vi"("error in"=w144, "data in"=w145, "Enum"=w130) -> ("error out"=w140:errorcluster)  [unwired: 5 in, 3 out]
        n70 = Type Cast(x=w138) -> (*(type *) &x=w137:string)  [unwired: 1 in]
        n71 = call "TCPIPmain.vi"("error in"=w140, "data in"=w137, "Enum"=w130) -> ("error out"=w139:errorcluster)  [unwired: 5 in, 3 out]
        n72 = Bundle By Name(cluster=w141, "Error"=w139) -> (w143:T2)
      }
      frame "DAQmx - Read" {
        # "/*读取原始振动数据*/"
        n73 = Unbundle By Name(w149) -> ("data out"=w148:T10)
        n74 = call "TCPIPmain.vi"("data"=w148, "Enum"=TCPIP_enum."read") -> ("error out"=w147:errorcluster, "data out"=w153:T10, "Data?"=w151:bool[])  [unwired: 6 in, 1 out]
        n75 = Or Array Elements(Boolean array=w151) -> (logical OR=w150:bool)
        n76 = case shown="真" w150 {
          tunnel: ["Idle" ("Remaining States") "DAQmx - Analyze" ("event")] -> w155
          frame False {
          }
          frame True {
          }
        }
        n77 = Bundle By Name(cluster=w149, "data out"=w153, "Error"=w147) -> (w152:T2)
      }
      frame "DAQmx - Analyze" {
        # "/*获取选中通道，并对选中的通道进行分析*/"
        n78 = Unbundle By Name(w162) -> ("data out"=w163:T10)
        n79 = call "CAL data.vi"("CAL"=T13 [{"T"={"TSlop"=[3004.15, 3004.15, 3004.15, 3004.15, 3004.15, 3004.15, 3004.15, 3004.15, 3004.15, 3004.15, 3004.15, 3004.15, 3004.15, 3004.15, 3004.15, 3004.15, 5631.89, 5631.89, 5631.89, 5631.89, 5631.89, 5631.89, 5631.89, 5631.89, 5631.89, 5631.89, 5631.89, 5631.89, 5631.89, 5631.89, 5631.89, 5631.89], "T0"=[-0.235, -0.469, -0.469, -0.469, -0.469, -0.469, -0.469, -0.469, -0.469, -0.469, -0.469, -0.469, -0.469, -0.469, -0.469, -0.469, -0.469, -0.469, -0.469, -0.469, -0.469, -0.469, -0.469, -0.469, -0.469, -0.469, -0.469, -0.469, -0.469, -0.469, -0.469, -0.235]}, "P"={"P0"=[-250.0, -250.0, -249.1, -250.0, -250.0, -250.0, -250.0, 0.0, 0.0, 0.0, 0.0, 0.0, 0.0, 0.0, 0.0, 0.0, -101.25, 0.0, 0.0, 0.0, -10.82, 0.0, 0.0, -145.23, 0.0, -250.0, -317.807, 0.0, 0.0, 0.0, 0.0, -145.23], "Pslop"=[150.0, 150.0, 127.525, 150.0, 150.0, 150.0, 150.0, 2500.0, 1.0, 1.0, 1.0, 1.0, 1.0, 1.0, 1.0, 1.0, 109.38, 1.0, 1.0, 1.0, 31.0966, 1.0, 1.0, 76.923, 1.0, 150.0, 152.074, 1.0, 1.0, 1.0, 1.0, 76.923]}}, {"T"={"TSlop"=[3004.15, 3004.15, 3004.15, 3004.15, 3004.15, 3004.15, 3004.15, 3004.15, 3004.15, 3004.15, 3004.15, 3004.15, 3004.15, 3004.15, 3004.15, 3004.15, 3004.15, 3004.15, 3004.15, 3004.15, 3004.15, 3004.15, 3004.15, 3004.15, 3004.15, 3004.15, 3004.15, 3004.15, 3004.15, 3004.15, 3004.15, 3004.15], "T0"=[-0.469, -0.469, -0.469, -0.469, -0.469, -0.469, -0.469, -0.469, -0.469, -0.469, -0.469, -0.469, -0.469, -0.469, -0.469, -0.469, -0.469, -0.469, -0.469, -0.469, -0.469, -0.469, -0.469, -0.469, -0.469, -0.469, -0.469, -0.469, -0.469, -0.469, -0.469, -0.469]}, "P"={"P0"=[-250.0, -250.0, -250.0, 0.0, 0.0, 0.0, 0.0, 0.0, -13.6259, 0.0, 0.0, -125.0, -250.0, 1.0, 1.0, 1.0, 0.0, -250.0, -250.0, -250.0, -250.0, 0.0, -250.0, -250.0, -250.0, 0.0, 0.0, 0.0, 0.0, 0.0, 0.0, 0.0], "Pslop"=[150.0, 150.0, 150.0, 1.0, 1.0, 1.0, 1.0, 2500.0, 26.4775, 1.0, 1.0, 125.0, 150.0, 1.0, 1.0, 1.0, 1.0, 150.0, 150.0, 150.0, 150.0, 1.0, 150.0, 150.0, 150.0, 1.0, 1.0, 1.0, 1.0, 1.0, 1.0, 1.0]}}, {"T"={"TSlop"=[3004.15, 3004.15, 3004.15, 3004.15, 3004.15, 3004.15, 3004.15, 3004.15, 3004.15, 3004.15, 3004.15, 3004.15, 3004.15, 3004.15, 3004.15, 3004.15, 5631.89, 5631.89, 5631.89, 5631.89, 5631.89, 5631.89, 5631.89, 5631.89, 5631.89, 5631.89, 5631.89, 5631.89, 5631.89, 5631.89, 5631.89, 5631.89], "T0"=[-0.235, -0.469, -0.469, -0.469, -0.469, -0.469, -0.469, -0.469, -0.469, -0.469, -0.469, -0.469, -0.469, -0.469, -0.469, -0.469, -0.469, -0.469, -0.469, -0.469, -0.469, -0.469, -0.469, -0.469, -0.469, -0.469, -0.469, -0.469, -0.469, -0.469, -0.469, -0.235]}, "P"={"P0"=[-250.0, -250.0, -249.1, -250.0, -250.0, -250.0, -250.0, 0.0, 0.0, 0.0, 0.0, 0.0, 0.0, 0.0, 0.0, 0.0, -101.25, 0.0, 0.0, 0.0, -10.82, 0.0, 0.0, -145.23, 0.0, -250.0, -317.807, 0.0, 0.0, 0.0, 0.0, -145.23], "Pslop"=[150.0, 150.0, 127.525, 150.0, 150.0, 150.0, 150.0, 2500.0, 1.0, 1.0, 1.0, 1.0, 1.0, 1.0, 1.0, 1.0, 109.38, 1.0, 1.0, 1.0, 31.0966, 1.0, 1.0, 76.923, 1.0, 150.0, 152.074, 1.0, 1.0, 1.0, 1.0, 76.923]}}, {"T"={"TSlop"=[3004.15, 3004.15, 3004.15, 3004.15, 3004.15, 3004.15, 3004.15, 3004.15, 3004.15, 3004.15, 3004.15, 3004.15, 3004.15, 3004.15, 3004.15, 3004.15, 3004.15, 3004.15, 3004.15, 3004.15, 3004.15, 3004.15, 3004.15, 3004.15, 3004.15, 3004.15, 3004.15, 3004.15, 3004.15, 3004.15, 3004.15, 3004.15], "T0"=[-0.469, -0.469, -0.469, -0.469, -0.469, -0.469, -0.469, -0.469, -0.469, -0.469, -0.469, -0.469, -0.469, -0.469, -0.469, -0.469, -0.469, -0.469, -0.469, -0.469, -0.469, -0.469, -0.469, -0.469, -0.469, -0.469, -0.469, -0.469, -0.469, -0.469, -0.469, -0.469]}, "P"={"P0"=[-250.0, -250.0, -250.0, 0.0, 0.0, 0.0, 0.0, 0.0, -13.6259, 0.0, 0.0, -125.0, -250.0, 1.0, 1.0, 1.0, 0.0, -250.0, -250.0, -250.0, -250.0, 0.0, -250.0, -250.0, -250.0, 0.0, 0.0, 0.0, 0.0, 0.0, 0.0, 0.0], "Pslop"=[150.0, 150.0, 150.0, 1.0, 1.0, 1.0, 1.0, 2500.0, 26.4775, 1.0, 1.0, 125.0, 150.0, 1.0, 1.0, 1.0, 1.0, 150.0, 150.0, 150.0, 150.0, 1.0, 150.0, 150.0, 150.0, 1.0, 1.0, 1.0, 1.0, 1.0, 1.0, 1.0]}}], "data out"=w163) -> ("CalData"=w159:T17)  [unwired: 9 in]
        n80 = call "cal formulate.vi"("CalData"=w159) -> ("caldataout"=w158:T17)  [unwired: 6 in]
        n81 = Bundle By Name(cluster=w162, "CalData"=w158) -> (w161:T2)
      }
      frame "DAQmx - Display" {
        # "/*显示分析结果*/"
        n82 = stacked-sequence {
          tunnel: ["DAQmx - Save Data" ("event") _ _ _ _ _ _ _ _ _] -> w166
          tunnel: w165 -> [w169 w176 w218 w241 w276 w320 w341 w363 w383 w414]
          frame #0 {
            n83 = Unbundle By Name(w169) -> ("CalData"=w170:T17)
            n84 = call "data to datatable.vi"("dis config Array"=T14 [{"T"=[{"index"=0.0, "name"="外回路温度", "unit"="℃", "代号"="T1"}, {"index"=1.0, "name"="外回路温度", "unit"="℃", "代号"="T2"}, {"index"=2.0, "name"="外回路温度", "unit"="℃", "代号"="T3"}, {"index"=3.0, "name"="外回路温度", "unit"="℃", "代号"="T4"}, {"index"=4.0, "name"="外回路温度", "unit"="℃", "代号"="PT1"}, {"index"=5.0, "name"="外回路温度", "unit"="℃", "代号"="PT2"}, {"index"=6.0, "name"="外回路温度", "unit"="℃", "代号"="PT3"}, {"index"=7.0, "name"="外回路温度", "unit"="℃", "代号"="Pt4"}, {"index"=8.0, "name"="外回路温度", "unit"="℃", "代号"="PT5"}, {"index"=10.0, "name"="外回路温度", "unit"="℃", "代号"="PT7"}, {"index"=11.0, "name"="外回路温度", "unit"="℃", "代号"="PT8"}, {"index"=12.0, "name"="外回路温度", "unit"="℃", "代号"="PT9"}, {"index"=9.0, "name"="外回路液温1", "unit"="℃", "代号"="PT6"}, {"index"=13.0, "name"="外回路液温2", "unit"="℃", "代号"="PT10"}], "P"=[{"index"=0.0, "name"="外回路压力", "unit"="Kpa", "代号"="P10"}, {"index"=1.0, "name"="外回路压力", "unit"="Kpa", "代号"="P11"}, {"index"=2.0, "name"="外回路压力", "unit"="Kpa", "代号"="P12"}, {"index"=3.0, "name"="外回路压力", "unit"="Kpa", "代号"="P13"}, {"index"=4.0, "name"="外回路压力", "unit"="Kpa", "代号"="P14"}, {"index"=5.0, "name"="外回路压力", "unit"="Kpa", "代号"="P15"}, {"index"=6.0, "name"="外回路压力", "unit"="Kpa", "代号"="P16"}, {"index"=7.0, "name"="外回路泵转速", "unit"="转/分", "代号"="转速"}, {"index"=20.0, "name"="外回路压差", "unit"="Kpa", "代号"=""}, {"index"=20.0, "name"="补偿器", "unit"="mm", "代号"="补偿器"}, {"index"=24.0, "name"="流量计", "unit"="L/H", "代号"="流量计"}, {"index"=25.0, "name"="外回路压力", "unit"="Kpa", "代号"="压力"}, {"index"=26.0, "name"="外回路压力", "unit"="Kpa", "代号"=""}, {"index"=31.0, "name"="温控阀角度", "unit"="度", "代号"="WKF1"}, {"index"=23.0, "name"="温控阀角度", "unit"="度", "代号"="WKF2"}], "state"=[{"index"=5.0, "name"="自锁阀状态", "unit"="", "代号"="ZSF1"}, {"index"=4.0, "name"="自锁阀状态", "unit"="", "代号"="ZSF2"}, {"index"=3.0, "name"="自锁阀状态", "unit"="", "代号"="ZSF3"}, {"index"=2.0, "name"="自锁阀状态", "unit"="", "代号"="ZSF4"}, {"index"=1.0, "name"="自锁阀状态", "unit"="", "代号"="ZSF5"}, {"index"=0.0, "name"="自锁阀状态", "unit"="", "代号"="ZSF6"}], "time"=timestamp(0 s since 1904-01-01), "targer"=enum."主舱外回路"}, {"T"=[{"index"=0.0, "name"="", "unit"="℃", "代号"="T1"}, {"index"=1.0, "name"="", "unit"="℃", "代号"="T2"}, {"index"=2.0, "name"="", "unit"="℃", "代号"="T3"}, {"index"=3.0, "name"="", "unit"="℃", "代号"="T4"}, {"index"=4.0, "name"="", "unit"="℃", "代号"="T5"}, {"index"=5.0, "name"="", "unit"="℃", "代号"="T6"}, {"index"=6.0, "name"="", "unit"="℃", "代号"="T7"}, {"index"=7.0, "name"="", "unit"="℃", "代号"="T8"}, {"index"=8.0, "name"="", "unit"="℃", "代号"="T9"}, {"index"=9.0, "name"="", "unit"="℃", "代号"="T10"}, {"index"=10.0, "name"="", "unit"="℃", "代号"="T11"}, {"index"=11.0, "name"="外回路液温1", "unit"="℃", "代号"="T12"}, {"index"=12.0, "name"="外回路液温2", "unit"="℃", "代号"="T13"}, {"index"=13.0, "name"="", "unit"="℃", "代号"="T14"}, {"index"=14.0, "name"="", "unit"="℃", "代号"="T15"}, {"index"=15.0, "name"="", "unit"="℃", "代号"="T16"}], "P"=[{"index"=0.0, "name"="", "unit"="Mpa", "代号"="P21"}, {"index"=1.0, "name"="", "unit"="Mpa", "代号"="P22"}, {"index"=2.0, "name"="", "unit"="Mpa", "代号"="P12"}, {"index"=8.0, "name"="", "unit"="V", "代号"="补偿器"}, {"index"=4.0, "name"="", "unit"="Mpa", "代号"="P14"}, {"index"=5.0, "name"="", "unit"="Mpa", "代号"="P15"}, {"index"=6.0, "name"="", "unit"="Mpa", "代号"="P16"}, {"index"=7.0, "name"="", "unit"="v", "代号"="泵转速"}, {"index"=8.0, "name"="", "unit"="Mpa", "代号"="P9"}, {"index"=9.0, "name"="P10", "unit"="Mpa", "代号"=""}, {"index"=10.0, "name"="", "unit"="Mpa", "代号"="P11"}, {"index"=11.0, "name"="", "unit"="Mpa", "代号"="P12"}, {"index"=12.0, "name"="", "unit"="Mpa", "代号"="P13"}, {"index"=13.0, "name"="", "unit"="v", "代号"="P14"}, {"index"=20.0, "name"="", "unit"="v", "代号"="补偿器"}, {"index"=24.0, "name"="", "unit"="v", "代号"="流量计"}, {"index"=25.0, "name"="压力", "unit"="Mpa", "代号"=""}, {"index"=26.0, "name"="压力", "unit"="Mpa", "代号"=""}], "state"=[{"index"=5.0, "name"="自锁阀状态", "unit"="", "代号"="ZSF7"}, {"index"=4.0, "name"="自锁阀状态", "unit"="", "代号"="ZSF8"}, {"index"=3.0, "name"="自锁阀状态", "unit"="", "代号"="ZSF9"}, {"index"=2.0, "name"="自锁阀状态", "unit"="", "代号"="ZSF10"}, {"index"=1.0, "name"="自锁阀状态", "unit"="", "代号"="ZSF11"}, {"index"=0.0, "name"="自锁阀状态", "unit"="", "代号"="ZSF12"}], "time"=timestamp(0 s since 1904-01-01), "targer"=enum."主舱外回路"}, {"T"=[{"index"=0.0, "name"="外回路温度", "unit"="℃", "代号"="T1"}, {"index"=1.0, "name"="外回路温度", "unit"="℃", "代号"="T2"}, {"index"=2.0, "name"="外回路温度", "unit"="℃", "代号"="T3"}, {"index"=3.0, "name"="外回路温度", "unit"="℃", "代号"="T4"}, {"index"=4.0, "name"="外回路温度", "unit"="℃", "代号"="PT1"}, {"index"=5.0, "name"="外回路温度", "unit"="℃", "代号"="PT2"}, {"index"=6.0, "name"="外回路温度", "unit"="℃", "代号"="PT3"}, {"index"=7.0, "name"="外回路温度", "unit"="℃", "代号"="Pt4"}, {"index"=8.0, "name"="外回路温度", "unit"="℃", "代号"="PT5"}, {"index"=10.0, "name"="外回路温度", "unit"="℃", "代号"="PT7"}, {"index"=11.0, "name"="外回路温度", "unit"="℃", "代号"="PT8"}, {"index"=12.0, "name"="外回路温度", "unit"="℃", "代号"="PT9"}, {"index"=9.0, "name"="外回路液温1", "unit"="℃", "代号"="PT6"}, {"index"=13.0, "name"="外回路液温2", "unit"="℃", "代号"="PT10"}], "P"=[{"index"=0.0, "name"="外回路压力", "unit"="Kpa", "代号"="P10"}, {"index"=1.0, "name"="外回路压力", "unit"="Kpa", "代号"="P11"}, {"index"=2.0, "name"="外回路压力", "unit"="Kpa", "代号"="P12"}, {"index"=3.0, "name"="外回路压力", "unit"="Kpa", "代号"="P13"}, {"index"=4.0, "name"="外回路压力", "unit"="Kpa", "代号"="P14"}, {"index"=5.0, "name"="外回路压力", "unit"="Kpa", "代号"="P15"}, {"index"=6.0, "name"="外回路压力", "unit"="Kpa", "代号"="P16"}, {"index"=7.0, "name"="外回路泵转速", "unit"="转/分", "代号"="转速"}, {"index"=20.0, "name"="外回路压差", "unit"="Kpa", "代号"=""}, {"index"=20.0, "name"="补偿器", "unit"="mm", "代号"="补偿器"}, {"index"=24.0, "name"="流量计", "unit"="L/H", "代号"="流量计"}, {"index"=25.0, "name"="外回路压力", "unit"="Kpa", "代号"="压力"}, {"index"=26.0, "name"="外回路压力", "unit"="Kpa", "代号"=""}, {"index"=31.0, "name"="温控阀角度", "unit"="度", "代号"="WKF1"}, {"index"=23.0, "name"="温控阀角度", "unit"="度", "代号"="WKF2"}], "state"=[{"index"=5.0, "name"="自锁阀状态", "unit"="", "代号"="ZSF1"}, {"index"=4.0, "name"="自锁阀状态", "unit"="", "代号"="ZSF2"}, {"index"=3.0, "name"="自锁阀状态", "unit"="", "代号"="ZSF3"}, {"index"=2.0, "name"="自锁阀状态", "unit"="", "代号"="ZSF4"}, {"index"=1.0, "name"="自锁阀状态", "unit"="", "代号"="ZSF5"}, {"index"=0.0, "name"="自锁阀状态", "unit"="", "代号"="ZSF6"}], "time"=timestamp(0 s since 1904-01-01), "targer"=enum."主舱外回路"}, {"T"=[{"index"=0.0, "name"="", "unit"="℃", "代号"="T1"}, {"index"=1.0, "name"="", "unit"="℃", "代号"="T2"}, {"index"=2.0, "name"="", "unit"="℃", "代号"="T3"}, {"index"=3.0, "name"="", "unit"="℃", "代号"="T4"}, {"index"=4.0, "name"="", "unit"="℃", "代号"="T5"}, {"index"=5.0, "name"="", "unit"="℃", "代号"="T6"}, {"index"=6.0, "name"="", "unit"="℃", "代号"="T7"}, {"index"=7.0, "name"="", "unit"="℃", "代号"="T8"}, {"index"=8.0, "name"="", "unit"="℃", "代号"="T9"}, {"index"=9.0, "name"="", "unit"="℃", "代号"="T10"}, {"index"=10.0, "name"="", "unit"="℃", "代号"="T11"}, {"index"=11.0, "name"="外回路液温1", "unit"="℃", "代号"="T12"}, {"index"=12.0, "name"="外回路液温2", "unit"="℃", "代号"="T13"}, {"index"=13.0, "name"="", "unit"="℃", "代号"="T14"}, {"index"=14.0, "name"="", "unit"="℃", "代号"="T15"}, {"index"=15.0, "name"="", "unit"="℃", "代号"="T16"}], "P"=[{"index"=0.0, "name"="", "unit"="Mpa", "代号"="P21"}, {"index"=1.0, "name"="", "unit"="Mpa", "代号"="P22"}, {"index"=2.0, "name"="", "unit"="Mpa", "代号"="P12"}, {"index"=8.0, "name"="", "unit"="V", "代号"="补偿器"}, {"index"=4.0, "name"="", "unit"="Mpa", "代号"="P14"}, {"index"=5.0, "name"="", "unit"="Mpa", "代号"="P15"}, {"index"=6.0, "name"="", "unit"="Mpa", "代号"="P16"}, {"index"=7.0, "name"="", "unit"="v", "代号"="泵转速"}, {"index"=8.0, "name"="", "unit"="Mpa", "代号"="P9"}, {"index"=9.0, "name"="P10", "unit"="Mpa", "代号"=""}, {"index"=10.0, "name"="", "unit"="Mpa", "代号"="P11"}, {"index"=11.0, "name"="", "unit"="Mpa", "代号"="P12"}, {"index"=12.0, "name"="", "unit"="Mpa", "代号"="P13"}, {"index"=13.0, "name"="", "unit"="v", "代号"="P14"}, {"index"=20.0, "name"="", "unit"="v", "代号"="补偿器"}, {"index"=24.0, "name"="", "unit"="v", "代号"="流量计"}, {"index"=25.0, "name"="压力", "unit"="Mpa", "代号"=""}, {"index"=26.0, "name"="压力", "unit"="Mpa", "代号"=""}], "state"=[{"index"=5.0, "name"="自锁阀状态", "unit"="", "代号"="ZSF7"}, {"index"=4.0, "name"="自锁阀状态", "unit"="", "代号"="ZSF8"}, {"index"=3.0, "name"="自锁阀状态", "unit"="", "代号"="ZSF9"}, {"index"=2.0, "name"="自锁阀状态", "unit"="", "代号"="ZSF10"}, {"index"=1.0, "name"="自锁阀状态", "unit"="", "代号"="ZSF11"}, {"index"=0.0, "name"="自锁阀状态", "unit"="", "代号"="ZSF12"}], "time"=timestamp(0 s since 1904-01-01), "targer"=enum."主舱外回路"}], "CalData"=w170) -> ("datatable"=→"测试数据":string[][])  [unwired: 9 in]
          }
          frame #1 {
            n85 = Unbundle By Name(w176) -> ("CalData"=w175:T17)
            n86 = call "find tagetdata.vi"("target"=enum16{"主舱外回路", "主舱内回路", "实验舱外回路", "实验舱内回路"}."主舱外回路", "CalData"=w175) -> ("data"=w174:T18, "find?"=w173:bool)  [unwired: 8 in]
            n87 = case shown="真" w173 {
              tunnel: w174 -> [_ w178]
              frame False {
              }
              frame True {
                n88 = Unbundle By Name(w178) -> ("P"=w189:dbl[], "time"=w177:timestamp)
                n89 = Index Array(array=w189, index #1=1 ("index"), index #2=2 ("index"), index #3=3 ("index"), index #4=4 ("index"), index #5=5 ("index"), index #6=6 ("index"), index #7=0 ("index"), index #8=16 ("index"), index #9=20 ("index"), index #10=24 ("index"), index #11=25 ("index"), index #12=26 ("index"), index #13=31 ("index"), index #14=23 ("index"), index #15=7 ("index")) -> (element #1=w185:dbl, element #2=w184:dbl, element #3=w183:dbl, element #4=w182:dbl, element #5=w181:dbl, element #6=→"P16":dbl, element #7=→"P10":dbl, element #8=→"DP1":dbl, element #9=→"补偿器":dbl, element #10=→"流量计":dbl, element #11=→"P34" →"P9":dbl, element #12=→"P35":dbl, element #13=→"wkf1" →"温控阀a":dbl, element #14=→"wkf2" →"温控阀ｂ":dbl, element #15=→"转速":dbl)
                "P11" <- w185
                "P12" <- w184
                "P13" <- w183
                "P14" <- w182
                "P15" <- w181
                n90 = Build Array(w185, w184, w183, w182, w181) -> (w180:dbl[])
                n91 = call "XY muliti ch chart.vi"("lenth"=2000, "clear?"=FALSE, "Data"=w180, "current time"=w177) -> ("XY Graph"=→"XY Graph":cluster{cluster{"time":dbl, "Y":dbl}[]}[])  [unwired: 7 in]
              }
            }
          }
          frame #2 {
            n92 = Unbundle By Name(w218) -> ("CalData"=w217:T17)
            n93 = call "find tagetdata.vi"("target"=enum16{"主舱外回路", "主舱内回路", "实验舱外回路", "实验舱内回路"}."主舱外回路", "CalData"=w217) -> ("data"=w215:T18, "find?"=w216:bool)  [unwired: 8 in]
            n94 = case shown="真" w216 {
              tunnel: w215 -> [_ w219]
              frame False {
              }
              frame True {
                n95 = Unbundle By Name(w219) -> ("tempt"=w220:dbl[])
                n96 = Index Array(array=w220, index #1=0 ("index"), index #2=1 ("index")) -> (element #1=→"T1":dbl, element #2=→"T2":dbl, element #3=→"T3":dbl, element #4=→"T4":dbl, element #5=→"PT1":dbl, element #6=→"PT2":dbl, element #7=→"PT3":dbl, element #8=→"PT4":dbl, element #9=→"PT5":dbl, element #10=→"temp1":dbl, element #11=→"PT7":dbl, element #12=→"PT8":dbl, element #13=→"PT9":dbl, element #14=→"temp2":dbl)  [unwired: 12 in]
              }
            }
          }
          frame #3 {
            n97 = Unbundle By Name(w241) -> ("CalData"=w240:T17)
            n98 = call "find tagetdata.vi"("target"=enum16{"主舱外回路", "主舱内回路", "实验舱外回路", "实验舱内回路"}."主舱内回路", "CalData"=w240) -> ("data"=w239:T18, "find?"=w238:bool)  [unwired: 8 in]
            n99 = case shown="真" w238 {
              tunnel: w239 -> [_ w242]
              frame False {
              }
              frame True {
                n100 = Unbundle By Name(w242) -> ("P"=w271:dbl[])
                n101 = Index Array(array=w271, index #1=16 ("index"), index #2=17 ("index"), index #3=18 ("index"), index #4=19 ("index"), index #5=20 ("index"), index #6=21 ("index"), index #7=22 ("index"), index #8=23 ("index"), index #9=8 ("index"), index #10=12 ("index"), index #11=7 ("index"), index #12=11 ("index"), index #13=0 ("index"), index #14=1 ("index")) -> (element #1=→"P14":dbl, element #2=→"P15":dbl, element #3=→"P16":dbl, element #4=→"P17":dbl, element #5=→"P18":dbl, element #6=→"流量计 2":dbl, element #7=→"P12":dbl, element #8=→"P13":dbl, element #9=→"补偿器":dbl, element #10=→"P19":dbl, element #11=→"转速":dbl, element #12=→"DP2":dbl, element #13=→"P10":dbl, element #14=→"P11":dbl)
              }
            }
          }
          frame #4 {
            n102 = Unbundle By Name(w276) -> ("CalData"=w275:T17)
            n103 = call "find tagetdata.vi"("target"=enum16{"主舱外回路", "主舱内回路", "实验舱外回路", "实验舱内回路"}."主舱内回路", "CalData"=w275) -> ("data"=w274:T18, "find?"=w273:bool)  [unwired: 8 in]
            n104 = case shown="真" w273 {
              tunnel: w274 -> [_ w277]
              frame False {
              }
              frame True {
                n105 = Unbundle By Name(w277) -> ("tempt"=w286:dbl[])
                n106 = Index Array(array=w286, index #1=20 ("index"), index #2=22 ("index"), index #3=19 ("index"), index #4=18 ("index"), index #5=21 ("index"), index #6=16 ("index"), index #7=17 ("index"), index #8=23 ("index")) -> (element #1=→"PT1":dbl, element #2=→"PT3":dbl, element #3=→"T4":dbl, element #4=→"T3":dbl, element #5=→"PT2":dbl, element #6=→"T1":dbl, element #7=→"T2":dbl, element #8=→"T22":dbl)
                n107 = Index Array(array=w286, index #1=0 ("index"), index #2=1 ("index"), index #3=2 ("index"), index #4=3 ("index")) -> (element #1=→"PT13":dbl, element #2=→"PT14":dbl, element #3=→"PT15":dbl, element #4=→"PT16":dbl)
                n108 = Index Array(array=w286, index #1=8 ("index"), index #2=9 ("index"), index #3=10 ("index"), index #4=12 ("index"), index #5=13 ("index")) -> (element #1=→"PT21":dbl, element #2=→"PT22":dbl, element #3=→"PT23":dbl, element #4=→"temp2 2":dbl, element #5=→"temp1 2":dbl)
              }
            }
          }
          frame #5 {
            n109 = Unbundle By Name(w320) -> ("CalData"=w319:T17)
            n110 = call "find tagetdata.vi"("target"=enum16{"主舱外回路", "主舱内回路", "实验舱外回路", "实验舱内回路"}."主舱外回路", "CalData"=w319) -> ("data"=w317:T18, "find?"=w316:bool)  [unwired: 8 in]
            n111 = call "find tagetdata.vi"("target"=enum16{"主舱外回路", "主舱内回路", "实验舱外回路", "实验舱内回路"}."主舱内回路", "CalData"=w319) -> ("data"=w318:T18, "find?"=w315:bool)  [unwired: 8 in]
            n112 = case shown="真" w316 {
              tunnel: w317 -> [_ w329]
              frame False {
              }
              frame True {
                n113 = Unbundle By Name(w329) -> ("state"=w336:bool[])
                n114 = Index Array(array=w336) -> (element #1=→"zsf6":bool, element #2=→"zsf5":bool, element #3=→"zsf4":bool, element #4=→"zsf3":bool, element #5=→"zsf2":bool, element #6=→"zsf1":bool)  [unwired: 6 in]
              }
            }
            n115 = case shown="真" w315 {
              tunnel: w318 -> [_ w321]
              frame False {
              }
              frame True {
                n116 = Unbundle By Name(w321) -> ("state"=w328:bool[])
                n117 = Index Array(array=w328) -> (element #1=→"zsf12":bool, element #2=→"zsf11":bool, element #3=→"zsf10":bool, element #4=→"zsf9":bool, element #5=→"zsf8":bool, element #6=→"zsf7":bool)  [unwired: 6 in]
              }
            }
          }
          frame #6 {
            n118 = Unbundle By Name(w341) -> ("CalData"=w340:T17)
            n119 = call "find tagetdata.vi"("target"=enum16{"主舱外回路", "主舱内回路", "实验舱外回路", "实验舱内回路"}."实验舱外回路", "CalData"=w340) -> ("data"=w339:T18, "find?"=w338:bool)  [unwired: 8 in]
            n120 = case shown="真" w338 {
              tunnel: w339 -> [_ w351]
              frame False {
              }
              frame True {
                n121 = Unbundle By Name(w351) -> ("P"=w358:dbl[])
                n122 = Index Array(array=w358, index #1=0 ("index"), index #2=6 ("index"), index #3=8 ("index"), index #4=9 ("index"), index #5=10 ("index")) -> (element #1=→"P10_syc":dbl, element #2=→"DP_syc":dbl, element #3=→"补偿器_sycw":dbl, element #4=→"syP9":dbl, element #5=→"syP35":dbl, element #6=→"实验舱温控阀a" →"wkf1 2":dbl, element #7=→"温控阀ｂ 2" →"wkf2 2":dbl, element #8=→"转速 2":dbl, element #9=→"电压 2":dbl, element #10=→"电流 2":dbl)  [unwired: 5 in]
              }
            }
          }
          frame #7 {
            n123 = Unbundle By Name(w363) -> ("CalData"=w362:T17)
            n124 = call "find tagetdata.vi"("target"=enum16{"主舱外回路", "主舱内回路", "实验舱外回路", "实验舱内回路"}."实验舱外回路", "CalData"=w362) -> ("data"=w361:T18, "find?"=w360:bool)  [unwired: 8 in]
            n125 = case shown="真" w360 {
              tunnel: w361 -> [_ w364]
              frame False {
              }
              frame True {
                n126 = Unbundle By Name(w364) -> ("tempt"=w378:dbl[])
                n127 = Index Array(array=w378) -> (element #1=→"T1_syc":dbl, element #2=→"PT7 2":dbl, element #3=→"PT9 2":dbl, element #4=→"PT5 2":dbl, element #5=→"temp2 3":dbl, element #6=→"temp1 3":dbl, element #7=→"PT4 2":dbl, element #8=→"T3 2":dbl, element #9=→"PT1 2":dbl, element #10=→"PT2 2":dbl, element #11=→"PT3 2":dbl, element #12=→"T2 2":dbl, element #13=→"PT8 2":dbl)  [unwired: 13 in]
              }
            }
          }
          frame #8 {
            n128 = Unbundle By Name(w383) -> ("CalData"=w382:T17)
            n129 = call "find tagetdata.vi"("target"=enum16{"主舱外回路", "主舱内回路", "实验舱外回路", "实验舱内回路"}."实验舱内回路", "CalData"=w382) -> ("data"=w380:T18, "find?"=w381:bool)  [unwired: 8 in]
            n130 = case shown="真" w381 {
              tunnel: w380 -> [_ w408]
              frame False {
              }
              frame True {
                n131 = Unbundle By Name(w408) -> ("P"=w409:dbl[])
                n132 = Index Array(array=w409, index #1=0 ("index"), index #2=1 ("index"), index #3=16 ("index"), index #4=19 ("index"), index #5=20 ("index"), index #6=24 ("index"), index #7=25 ("index"), index #8=26 ("index"), index #9=27 ("index"), index #10=28 ("index"), index #11=29 ("index"), index #12=30 ("index")) -> (element #1=→"P10 3":dbl, element #2=→"P11 3":dbl, element #3=→"补偿器 2":dbl, element #4=→"DP2 2":dbl, element #5=→"P19syc":dbl, element #6=→"P14 3":dbl, element #7=→"P15 3":dbl, element #8=→"P16 3":dbl, element #9=→"P17 2":dbl, element #10=→"P18 2":dbl, element #11=→"P13 3":dbl, element #12=→"P12 3":dbl)  [unwired: 1 in, 1 out]
              }
            }
          }
          frame #9 {
            n133 = Unbundle By Name(w414) -> ("CalData"=w413:T17)
            n134 = call "find tagetdata.vi"("target"=enum16{"主舱外回路", "主舱内回路", "实验舱外回路", "实验舱内回路"}."实验舱内回路", "CalData"=w413) -> ("data"=w412:T18, "find?"=w411:bool)  [unwired: 8 in]
            n135 = case shown="真" w411 {
              tunnel: w412 -> [_ w416]
              frame False {
              }
              frame True {
                n136 = Unbundle By Name(w416) -> ("tempt"=w434:dbl[])
                n137 = Index Array(array=w434) -> (element #1=→"PT1 3":dbl, element #2=→"T4 2":dbl, element #3=→"PT2 3":dbl, element #4=→"PT3 3":dbl, element #5=→"T3 3":dbl, element #6=→"T1 3":dbl, element #7=→"T2 3":dbl, element #8=→"T22 2":dbl, element #9=→"temp2 4":dbl, element #10=→"temp1 4":dbl, element #11=→"PT22 2":dbl, element #12=→"PT21 2":dbl, element #13=→"PT23 2":dbl, element #14=→"PT13 2":dbl, element #15=→"PT14 2":dbl, element #16=→"PT15 2":dbl, element #17=→"PT16 2":dbl, element #18=→"T4 3":dbl)  [unwired: 18 in]
              }
            }
          }
        }
      }
      frame "DAQmx - Save Data" {
        n138 = disable-structure shown="Disabled" {
          disable-tunnel: w436 -> [w437 _]
          frame Disabled {
            # "/*保存振动数据*/"
            n139 = Unbundle By Name(w437) -> ("Error"=w438:errorcluster)
            n140 = call "trigier.vi"("enum"=T15."trig") -> ("triger?"=→"triger?":bool, "save?"=w439:bool)  [unwired: 3 in, 6 out]
            "save" <- w439
            n141 = case shown="真" w439 {
              tunnel: w438 -> [w442 w444]
              tunnel: [w442 w444] -> _
              frame False {
                (unwired) u8 0 ("禁用")
                n142 = local write "save"(FALSE) -> ()
              }
              frame True {
                n143 = local write "save"(TRUE) -> ()
              }
            }
          }
          frame Enabled {
          }
        }
      }
      frame "DAQmx - Clear" {
        w449 = T1 12 items=["NO_Action", "start", "pause", "resum", "stop", "config", "System_constant", "7", "DAQ_init", "DAQ_config", "DAQ_start", "DAQ_read", "DAQ_stop", "DAQ_contrl", "14", "15", "16", "17", "18", "19", ""] ("command")
        (unwired) u8 2 ("禁用")
        (unwired) FALSE ("save")
        # "/*清除任务，关闭文件，清空队列*/"
        n144 = Unbundle By Name(w451) -> ("Error"=w453:errorcluster)
        n145 = call "File IO - FGV(V)_SubVIs-某型振动实验台测试系统.vi"("error in"=w453, "Operation"=Enum_File_IO_-_FGV(V)_Ctrls-某型振动实验台测试系统."Close") -> ("error out"=w458:errorcluster)  [unwired: 8 in, 9 out]
        n146 = call "Event Queues Manager_SubVIs-某型振动实验台测试系统.vi"("Mode"=Enum_queue_Ctrls-某型振动实验台测试系统."Flush Pro1" ("Mod"), "error in"=w458) -> ("error out"=w448:errorcluster)  [unwired: 3 in, 6 out]
        n147 = local write "Acquire"(FALSE ("Acquire")) -> ()
        n148 = Type Cast(x=w449) -> (*(type *) &x=w450:string)  [unwired: 1 in]
        n149 = call "TCPIPmain.vi"("error in"=w448, "data in"=w450, "Enum"=TCPIP_enum."write") -> ("error out"=w446:errorcluster)  [unwired: 5 in, 3 out]
        n150 = Bundle By Name(cluster=w451, "StateName"="Normal", "Error"=w446) -> (w457:T2)
      }
      frame "---------------------" {
      }
      frame "Error Handle" {
        # "/*若发生错误，进行错误处理*/"
        n151 = Unbundle By Name(w466) -> ("Error"=w464:errorcluster)
        n152 = call "Error Handle_SubVIs-某型振动实验台测试系统.vi"("error in"=w464) -> ("error out"=w463:errorcluster)  [unwired: 10 out]
        n153 = Bundle By Name(cluster=w466, "Error"=w463) -> (w465:T2)
      }
      frame "About" {
        n154 = Unbundle By Name(w471) -> ("Error"=w468:errorcluster)
        n155 = call "About.vi"("error in (no error)"=w468) -> ("error out"=w467:errorcluster)  [unwired: 10 out]
        n156 = Bundle By Name(cluster=w471, "Error"=w467) -> (w470:T2)
      }
      frame "Exit" {
        n157 = Unbundle By Name(w474) -> ("Error"=w476:errorcluster)
        n158 = call "Event Queues Manager_SubVIs-某型振动实验台测试系统.vi"("Mode"=Enum_queue_Ctrls-某型振动实验台测试系统."Destroy Pro1" ("Mod"), "error in"=w476) -> ("error out"=w475:errorcluster)  [unwired: 3 in, 6 out]
        n159 = Bundle By Name(cluster=w474, "Error"=w475) -> (w473:T2)
        n160 = disable-structure shown="Enabled" {
          frame Disabled {
            n161 = Quit LabVIEW(quit? (T)=TRUE) -> ()
          }
          frame Enabled {
          }
        }
      }
    }
  }
  n162 = while {
    shift-right: [w482] -> _
    shift-left: w1 -> [w483]
    stop <- w480 stop-if-true
    n163 = event shown="[4] \"ZP\", \"WP\": 值改变" {
      selector: _ -> [_ _ _ _ _ _ _ _ _ _ _ _]
      dyn-events: _ -> [_ _ _ _ _ _ _ _ _ _ _ _]
      timeout: 10 -> [_ _ _ _ _ _ _ _ _ _ _ _]
      tunnel: w483 -> [w484 w490 w495 w506 w516 _ w534 w550 w582 w608 w641 w646]
      tunnel: [w485 w489 w494 w505 w515 _ _ w551 w581 w607 w640 w645] -> w482
      tunnel: [_ _ w493 _ _ _ _ _ _ _ _ TRUE] -> w480
      event Timeout {
        # "/*判断是否有错误发生，若有错误发生，\n进入错误处理状态*/"
        n164 = event-data() -> ()  [unwired: 3 out]
        n165 = case shown="无错误" w484 {
          selector: w484 -> [w486 w487]
          tunnel: [w486 w488] -> w485
          frame No Error {
          }
          frame Error {
            n166 = call "Error Handle_SubVIs-某型振动实验台测试系统.vi"("error in"=w487) -> ("error out"=w488:errorcluster)  [unwired: 10 out]
          }
        }
      }
      event "Config": Value Change {
        # "/*若配置键被按下，进入到配置状态中*/"
        n167 = event-data() -> ()  [unwired: 2 out]
        n168 = call "Event Queues Manager_SubVIs-某型振动实验台测试系统.vi"("Mode"=Enum_queue_Ctrls-某型振动实验台测试系统."Send Pro1" ("Mod"), "error in"=w490, "event"="Configurate") -> ("error out"=w489:errorcluster)  [unwired: 2 in, 6 out]
      }
      event Menu Selection (User) {
        # "/*按照选中的菜单标签跳转到相应状态*/"
        n169 = event-data() -> ("ItemTag"=w496:string)  [unwired: 1 out]
        n170 = case shown="\"Help - About\"" w496 {
          tunnel: [_ "Configurate" ("event") "Exit" ("event") "Input Test Name" ("event") "Query" ("event") "About" ("event")] -> w498
          tunnel: [_ _ TRUE _ _ _] -> w493
          frame "", Default {
          }
          frame "File - Configure" {
          }
          frame "Exit" {
          }
          frame "Operate - Run" {
          }
          frame "Operate - Query" {
          }
          frame "Help - About" {
          }
        }
        n171 = call "Event Queues Manager_SubVIs-某型振动实验台测试系统.vi"("Mode"=Enum_queue_Ctrls-某型振动实验台测试系统."Send Pro1" ("Mod"), "error in"=w495, "event"=w498) -> ("error out"=w494:errorcluster)  [unwired: 2 in, 6 out]
      }
      event "Acquire": Value Change {
        n172 = event-data() -> ("NewVal"=w511:bool)  [unwired: 1 out]
        n173 = Select(t="Input Test Name" ("event"), s=w511, f="DAQmx - Clear" ("event")) -> (s? t:f=w507:string)
        n174 = call "Event Queues Manager_SubVIs-某型振动实验台测试系统.vi"("Mode"=Enum_queue_Ctrls-某型振动实验台测试系统."Send Pro1" ("Mod"), "error in"=w506, "event"=w507) -> ("error out"=w505:errorcluster)  [unwired: 2 in, 6 out]
      }
      event "ZP", "WP": Value Change {
        w519 = T1 23 items=["NO_Action", "start", "pause", "resum", "stop", "config", "System_constant", "7", "DAQ_init", "DAQ_config", "DAQ_start", "DAQ_read", "DAQ_stop", "DAQ_contrl", "14", "15", "16", "17", "18", "19", "Zsf_open", "Zsf_close", "Wkf_control", "Pump_switch", "dcf_switch", "JRQ_switch"] ("command")
        n175 = event-data() -> ("CtlRef"=w514:refnum<vi>, "NewVal"=w528:bool)  [unwired: 1 out]
        n176 = control-ref of="WP"() -> (w513:refnum<vi>)
        n177 = control-ref of="ZP"() -> (w512:refnum<vi>)
        n178 = Build Array(w513, w512) -> (w529:refnum<vi>[])
        n179 = Search 1D Array(1D array=w529, element=w514) -> (index of element=w521:i32)  [unwired: 1 in]
        n180 = To Unsigned Word Integer(number=w521) -> (unsigned 16bit integer=w520:u16)
        n181 = Boolean To (0,1)(Boolean=w528) -> (0, 1=w527:i16)
        n182 = To Unsigned Byte Integer(number=w527) -> (unsigned 8bit integer=w526:u8)
        n183 = Type Cast(x=w526) -> (*(type *) &x=w524:string)  [unwired: 1 in]
        n184 = Type Cast(x=w519) -> (*(type *) &x=w525:string)  [unwired: 1 in]
        n185 = Concatenate Strings(w525, w524) -> (w522:string)
        n186 = Type Cast(type=enum16{"主舱外回路", "主舱内回路", "实验舱外回路", "实验舱内回路"}."主舱外回路" ("targer"), x=w520) -> (*(type *) &x=w517:enum16{"主舱外回路", "主舱内回路", "实验舱外回路", "实验舱内回路"})
        n187 = call "TCPIPmain.vi"("error in"=w516, "data in"=w522, "targer"=w517, "Enum"=TCPIP_enum."command") -> ("error out"=w515:errorcluster)  [unwired: 4 in, 3 out]
      }
      event "temctr_type": Value Change {
        n188 = event-data() -> ("NewVal"=w531:enum16{"开度", "控温"})  [unwired: 3 out]
        n189 = case shown="\"控温\"" w531 {
          tunnel: ["°" "℃"] -> w530
          frame "开度", Default {
          }
          frame "控温" {
          }
        }
        "unit" <- w530
      }
      event "temctr_run": Value Change {
        n190 = event-data() -> ("NewVal"=w535:bool)  [unwired: 1 out]
        n191 = case shown="真" w535 {
          tunnel: w534 -> [_ w546]
          frame False {
          }
          frame True {
            w544 = T1 22 items=["NO_Action", "start", "pause", "resum", "stop", "config", "System_constant", "7", "DAQ_init", "DAQ_config", "DAQ_start", "DAQ_read", "DAQ_stop", "DAQ_contrl", "14", "15", "16", "17", "18", "19", "Zsf_open", "Zsf_close", "Wkf_control", "Pump_switch", "dcf_switch", "JRQ_switch"] ("command")
            n192 = To Unsigned Byte Integer(number="temctr_type") -> (unsigned 8bit integer=w536:u8)
            n193 = Type Cast(x=w544) -> (*(type *) &x=w547:string)  [unwired: 1 in]
            n194 = To Unsigned Byte Integer(number=u8 0) -> (unsigned 8bit integer=w537:u8)
            n195 = Type Cast(x="temctr_value") -> (*(type *) &x=w541:string)  [unwired: 1 in]
            n196 = Type Cast(x=w536) -> (*(type *) &x=w539:string)  [unwired: 1 in]
            n197 = Type Cast(x=w537) -> (*(type *) &x=w540:string)  [unwired: 1 in]
            n198 = Concatenate Strings(w547, w539, w540, w541) -> (w549:string)
            n199 = call "TCPIPmain.vi"("error in"=w546, "data in"=w549, "targer"=enum16{"主舱外回路", "主舱内回路", "实验舱外回路", "实验舱内回路"}."主舱外回路", "Enum"=TCPIP_enum."command") -> ()  [unwired: 4 in, 4 out]
          }
        }
      }
      event "temctr_run 2": Value Change {
        n200 = event-data() -> ("NewVal"=w552:bool)  [unwired: 1 out]
        n201 = case shown="真" w552 {
          tunnel: [w553 w562] -> w551
          tunnel: w550 -> [w553 w561]
          frame False {
          }
          frame True {
            w564 = T1 22 items=["NO_Action", "start", "pause", "resum", "stop", "config", "System_constant", "7", "DAQ_init", "DAQ_config", "DAQ_start", "DAQ_read", "DAQ_stop", "DAQ_contrl", "14", "15", "16", "17", "18", "19", "Zsf_open", "Zsf_close", "Wkf_control", "Pump_switch", "dcf_switch", "JRQ_switch"] ("command")
            n202 = To Unsigned Byte Integer(number="temctr_type 2") -> (unsigned 8bit integer=w555:u8)
            n203 = To Unsigned Byte Integer(number=u8 1) -> (unsigned 8bit integer=w554:u8)
            n204 = Type Cast(x=w555) -> (*(type *) &x=w558:string)  [unwired: 1 in]
            n205 = Type Cast(x=w564) -> (*(type *) &x=w566:string)  [unwired: 1 in]
            n206 = Type Cast(x="temctr_value 2") -> (*(type *) &x=w563:string)  [unwired: 1 in]
            n207 = Type Cast(x=w554) -> (*(type *) &x=w559:string)  [unwired: 1 in]
            n208 = Concatenate Strings(w566, w558, w559, w563) -> (w568:string)
            n209 = call "TCPIPmain.vi"("error in"=w561, "data in"=w568, "targer"=enum16{"主舱外回路", "主舱内回路", "实验舱外回路", "实验舱内回路"}."主舱外回路", "Enum"=TCPIP_enum."command") -> ("error out"=w562:errorcluster)  [unwired: 4 in, 3 out]
          }
        }
      }
      event "ZSF01", "ZSF02", "ZSF03", "ZSF04", "ZSF05", "ZSF06", "ZSF07", "ZSF08", "ZSF09", "ZSF10", "ZSF11", "ZSF12": Value Change {
        w576 = T1 21 items=["NO_Action", "start", "pause", "resum", "stop", "config", "System_constant", "7", "DAQ_init", "DAQ_config", "DAQ_start", "DAQ_read", "DAQ_stop", "DAQ_contrl", "14", "15", "16", "17", "18", "19", "Zsf_open", "Zsf_close", "Wkf_control", "Pump_switch", "dcf_switch", "JRQ_switch"] ("command")
        w577 = T1 20 items=["NO_Action", "start", "pause", "resum", "stop", "config", "System_constant", "7", "DAQ_init", "DAQ_config", "DAQ_start", "DAQ_read", "DAQ_stop", "DAQ_contrl", "14", "15", "16", "17", "18", "19", "Zsf_open", "Zsf_close", "Wkf_control", "Pump_switch", "dcf_switch", "JRQ_switch"] ("command")
        n210 = event-data() -> ("CtlRef"=w583:refnum<vi>, "NewVal"=w575:bool)  [unwired: 1 out]
        n211 = control-ref of="ZSF08"() -> (w589:refnum<vi>)
        n212 = control-ref of="ZSF01"() -> (w596:refnum<vi>)
        n213 = control-ref of="ZSF02"() -> (w595:refnum<vi>)
        n214 = control-ref of="ZSF03"() -> (w594:refnum<vi>)
        n215 = control-ref of="ZSF04"() -> (w593:refnum<vi>)
        n216 = control-ref of="ZSF05"() -> (w592:refnum<vi>)
        n217 = control-ref of="ZSF06"() -> (w591:refnum<vi>)
        n218 = control-ref of="ZSF07"() -> (w590:refnum<vi>)
        n219 = control-ref of="ZSF10"() -> (w587:refnum<vi>)
        n220 = control-ref of="ZSF11"() -> (w586:refnum<vi>)
        n221 = control-ref of="ZSF12"() -> (w585:refnum<vi>)
        n222 = control-ref of="ZSF09"() -> (w588:refnum<vi>)
        n223 = Build Array(w596, w595, w594, w593, w592, w591, w590, w589, w588, w587, w586, w585) -> (w584:refnum<vi>[])
        n224 = Search 1D Array(1D array=w584, element=w583) -> (index of element=w573:i32)  [unwired: 1 in]
        n225 = case shown="6..12" w573 {
          selector: w573 -> [w598 w600 w604]
          tunnel: [w598 w600 w602] -> w570
          tunnel: [enum16{"主舱外回路", "主舱内回路", "实验舱外回路", "实验舱内回路"}."主舱外回路" ("targer") enum16{"主舱外回路", "主舱内回路", "实验舱外回路", "实验舱内回路"}."主舱外回路" ("targer") enum16{"主舱外回路", "主舱内回路", "实验舱外回路", "实验舱内回路"}."主舱内回路" ("targer")] -> w569
          frame 0..5 {
          }
          frame 16, Default {
          }
          frame 6..12 {
            n226 = Subtract(x=w604, y=6) -> (x-y=w602:i32)
          }
        }
        n227 = Select(t=w577, s=w575, f=w576) -> (s? t:f=w578:T1)
        n228 = Type Cast(x=w578) -> (*(type *) &x=w574:string)  [unwired: 1 in]
        n229 = To Unsigned Byte Integer(number=w570) -> (unsigned 8bit integer=w572:u8)
        n230 = Type Cast(x=w572) -> (*(type *) &x=w571:string)  [unwired: 1 in]
        n231 = Concatenate Strings(w574, w571) -> (w580:string)
        n232 = call "TCPIPmain.vi"("error in"=w582, "data in"=w580, "targer"=w569, "Enum"=TCPIP_enum."command") -> ("error out"=w581:errorcluster)  [unwired: 4 in, 3 out]
      }
      event "DCF1", "DCF2", "DCF3", "DCF4", "DCF5", "DCF6", "DCF8", "DCF9", "DCF10", "DCF11", "DCF12", "DCF13", "DCF14", "DCF15", "DCF16", "DCF17", "DCF18", "DCF19", "DCF7": Value Change {
        w617 = T1 24 items=["NO_Action", "start", "pause", "resum", "stop", "config", "System_constant", "7", "DAQ_init", "DAQ_config", "DAQ_start", "DAQ_read", "DAQ_stop", "DAQ_contrl", "14", "15", "16", "17", "18", "19", "Zsf_open", "Zsf_close", "Wkf_control", "Pump_switch", "dcf_switch", "JRQ_switch"] ("command")
        n233 = event-data() -> ("CtlRef"=w605:refnum<vi>, "NewVal"=w615:bool)  [unwired: 1 out]
        n234 = control-ref of="DCF7"() -> (w633:refnum<vi>)
        n235 = control-ref of="DCF8"() -> (w632:refnum<vi>)
        n236 = control-ref of="DCF9"() -> (w631:refnum<vi>)
        n237 = control-ref of="DCF10"() -> (w630:refnum<vi>)
        n238 = control-ref of="DCF11"() -> (w629:refnum<vi>)
        n239 = control-ref of="DCF12"() -> (w628:refnum<vi>)
        n240 = control-ref of="DCF13"() -> (w627:refnum<vi>)
        n241 = control-ref of="DCF14"() -> (w626:refnum<vi>)
        n242 = control-ref of="DCF15"() -> (w625:refnum<vi>)
        n243 = control-ref of="DCF16"() -> (w624:refnum<vi>)
        n244 = control-ref of="DCF17"() -> (w623:refnum<vi>)
        n245 = control-ref of="DCF18"() -> (w622:refnum<vi>)
        n246 = control-ref of="DCF19"() -> (w621:refnum<vi>)
        n247 = control-ref of="DCF1"() -> (w639:refnum<vi>)
        n248 = control-ref of="DCF2"() -> (w638:refnum<vi>)
        n249 = control-ref of="DCF3"() -> (w637:refnum<vi>)
        n250 = control-ref of="DCF4"() -> (w636:refnum<vi>)
        n251 = control-ref of="DCF5"() -> (w635:refnum<vi>)
        n252 = control-ref of="DCF6"() -> (w634:refnum<vi>)
        n253 = Build Array(w639, w638, w637, w636, w635, w634, w633, w632, w631, w630, w629, w628, w627, w626, w625, w624, w623, w622, w621) -> (w620:refnum<vi>[])
        n254 = Search 1D Array(1D array=w620, element=w605) -> (index of element=w619:i32)  [unwired: 1 in]
        n255 = Boolean To (0,1)(Boolean=w615) -> (0, 1=w616:i16)
        n256 = To Unsigned Byte Integer(number=w619) -> (unsigned 8bit integer=w618:u8)
        n257 = To Unsigned Byte Integer(number=w616) -> (unsigned 8bit integer=w614:u8)
        n258 = Type Cast(x=w617) -> (*(type *) &x=w606:string)  [unwired: 1 in]
        n259 = Type Cast(x=w614) -> (*(type *) &x=w612:string)  [unwired: 1 in]
        n260 = Type Cast(x=w618) -> (*(type *) &x=w613:string)  [unwired: 1 in]
        n261 = Concatenate Strings(w606, w613, w612) -> (w610:string)
        n262 = call "TCPIPmain.vi"("error in"=w608, "data in"=w610, "targer"=enum16{"主舱外回路", "主舱内回路", "实验舱外回路", "实验舱内回路"}."主舱内回路", "Enum"=TCPIP_enum."command") -> ("error out"=w607:errorcluster)  [unwired: 4 in, 3 out]
      }
      event "Query": Value Change {
        n263 = event-data() -> ()  [unwired: 2 out]
        n264 = call "Event Queues Manager_SubVIs-某型振动实验台测试系统.vi"("Mode"=Enum_queue_Ctrls-某型振动实验台测试系统."Send Pro1" ("Mod"), "error in"=w641, "event"="Query") -> ("error out"=w640:errorcluster)  [unwired: 2 in, 6 out]
      }
      event "Exit": Value Change {
        n265 = event-data() -> ()  [unwired: 2 out]
        n266 = call "Event Queues Manager_SubVIs-某型振动实验台测试系统.vi"("Mode"=Enum_queue_Ctrls-某型振动实验台测试系统."Send Pro1" ("Mod"), "error in"=w646, "event"="Exit") -> ("error out"=w645:errorcluster)  [unwired: 2 in, 6 out]
      }
    }
  }
